vi "TOP LEVEL VI.vi"() -> ()   [LabVIEW 2020]
doc: "This Continuous Measurement sample project is based on the Queued Message Handler template.\n\nThe Event Handling Loop generates messages based on user interface actions.\n\nThe Message Handling Loop processes messages generated by the Event Handling Loop, or by other messages. There are also Acquisition and Logging message handling loop subVIs, and a chart updating loop."
uses:
  Typedefs/Objective selector control enum.ctl
  Typedefs/Laser control knob.ctl
  Typedefs/PMT control knob.ctl
  Typedefs/Frame Size.ctl
  Typedefs/AOL modes.ctl
  Peripherals Control/XYZ Stage/Typedefs/XYZ channel ring.ctl
  Typedefs/Plane Mode.ctl
  Typedefs/AVI implementation enum.ctl
  Acquisition/Typedefs/Ref DAQ Param.ctl
  Typedefs/XY Stage_Move.ctl
  Typedefs/test_fpga_control.ctl
  Typedefs/Reference source.ctl
  User Interface/Typedefs/Laser 1 switch.ctl
  User Interface/Misc/Biology Information.ctl
  User Interface/Misc/Experiment Type.ctl
  Peripherals Control/Laser Ops (Generic)/Type Defs/Ls1 wav cancel.ctl
  Typedefs/Low-High Resolution Settings.ctl
  Typedefs/UI ctrl refs cluster.ctl
  User Interface/Typedefs/Next state queue data.ctl
  Typedefs/Start-Stop Enum.ctl
  Typedefs/Top level VI states.ctl
  Typedefs/Shutter Function Enum.ctl
  <vilib>/Utility/error.llb/DialogType.ctl
  Peripherals Control/Laser Ops (Generic)/Type Defs/Ls1 User Ops.ctl
  Typedefs/fgv_actions.ctl
  Logging/Globals/gl_Binary time series files globals.vi
  Peripherals Control/Pockels/Globals/gl_Pockels control globals.vi
  Global Variables/General Globals.vi
  Peripherals Control/XYZ Stage/Globals/gl_XYZStage globals.vi
  Global Variables/gl_UI Ctrl Refs.vi
  Peripherals Control/XYZ Stage/Typedefs/XYZ stage states.ctl
  Peripherals Control/XYZ Stage/Typedefs/XYZ stage data.ctl
panel:
  out "Camera recording status":bool
  out "Ls1 Status Ind":T1
  in  "Motor Z Stack":bool
  in  "AOL Z Stack":bool
  in  "Live Imaging":bool
  in  "Speed Logging":bool
  in  "Time Lapse":bool
  out "Ls1 wav top Ind":string caption="LASER wavelength"
  out "Ls1 power top Ind":string caption="LASER Output Power"
  in  "Dummy button":bool
  in  "Motor E-Stop":bool
  in  "Movement Correction":bool
  in  "Axis":T2="All" caption="Axis to zero"
  in  "Set as Origin":bool
  out "Stage XYZ Position":cluster{"X":sgl, "Y":sgl, "Z":sgl} caption="Current Stage Position (µm)" {"Z" format="Z:%#_g"; "Y" format="Y:%#_g"; "X" format="X:%#_g"}
  out "Stop":bool=TRUE
  in  "AOL Mode":T3
  in  "Frame Size":T4=512 items=["100X100"=100, "128X128"=128, "200X200"=200, "256X256"=256, "512X512"=512, "1024x1024"=1024, "2048x2048"=2048]
  in  "Objective":T5="Olympus  20X"
  in  "Funct Acq button":bool
  in  "Exit button":bool
  in  "Imaging Param Tab":T6(tab)
  in  "Field of View":sgl(slide)=100.0 min=100 max=500 step=5 scale=100.0..500.0
  in  "AOL Z":sgl(slide) min=-113.4277 max=113.4277 step=0.01 scale=-113.42766999434922..113.42766999434922 scale format="%#_2f"
  in  "PMT 1":T7 max=1000 step=5 scale=0.0..1000.0
  in  "PMT 2":T7 max=1000 step=5 scale=0.0..1000.0
  in  "Zoom":i8(slide)=1 min=1 max=24 step=1 scale=1.0..24.0
  out "Back aperture power (ind.)":dbl format="%#.0fmW"
  in  "Laser Power":T8 caption="LASER" max=1000 step=1 scale=0.0..100.0 scale format="%.0f%"
  out "Power after objective (ind.)":dbl format="%#.0fmW"
  in  "Averages":u16(knob) max=16 step=1 scale=0.0..16.0
  out "Ls1 Note":string
  in  "Dwell Time":dbl=0.10000000149011612 min=0.05 max=12.0 step=0.05000000074505806 format="%#.2fµs"
  in  "Optimise Obj. Pos.":bool=TRUE caption="Optimise Objective Position for AOL Z-stack"
  in  "Obtain Z Stop":bool
  in  "Obtain Z Start":bool
  in  "# Planes":u16=21 min=1 max=1000
  in  "Pockels@Z Stop":u16=5 caption="Laser % at Z Stop" max=100 format="%.0f%"
  in  "Pockels@Z Start":u16=5 caption="Laser % at Z Start" max=100 format="%.0f%"
  in  "Z Step":dbl=2.0 min=0.1 max=500.0 step=0.1 format="%#.1fµm"
  in  "Z Stop":dbl=-25.0 step=1.0 format="%#.0fµm"
  in  "Z Start":dbl=25.0 step=1.0 format="%#.0fµm"
  in  "Ls1 wav cancel":T9
  out "Ls1 Pump peak Hold":bool caption="Laser Pump peak Hold"
  in  "Ls1 Wavelength":dbl caption="Wavelength" format="%#_g [nm]"
  in  "Ls1 Confirm Wav":bool
  out "Ls1 PreChrp Prism2":dbl
  out "Ls1 PreChrp Prism1":dbl caption="Prechirper Prism 1"
  out "Ls1Tuning Status":string caption="Tuning Status"
  out "Ls1 Conn. Status":string caption="Laser Conn. Status"
  out "Ls1 Faults":string caption="Faults"
  out "Ls1 Mode":string caption="Mode"
  in  "Ls1Shutter":bool
  out "Ls1 POWER [mW]":dbl caption="Laser POWER [mW]"
  in  "Hard Shutter":bool
  in  "Virtual Shutter":bool
  out "Center freq ind (nm)":dbl caption="Center frequency" min=800.0 max=1080.0 step=1.0 format="%#.2f MHz"
  out "Ls1 Connection":bool
  in  "Enable f.acq post-processing":bool=TRUE
  in  "Video Record-Funct acq":bool
  in  "Video Record-Live Imaging":bool
  in  "Enable Video Recording":bool
  in  "Plane Mode":T10 items=["XY Plane", "XZ Plane", "YZ Plane", "arbitraryplane"]
  in  "Angle (degrees)":dbl caption="Angle" min=-180.0 max=180.0 format="%#_g°"
  in  "Y centre":dbl min=-1.0 max=1.0 step=0.1 format="%#.2f"
  in  "X centre":dbl min=-1.0 max=1.0 step=0.1 format="%#.2f"
  in  "Live stim.trig.period":dbl=10.0 caption="Stimulus trigger period" min=0.001 max=50.0 step=1.0 format="%#.6f s"
  in  "Live stim.trig.enable":bool caption="Enable stimulus"
  in  "Show ref plots window":bool
  in  "XY Stage Move":T11={"Move"=enum."y_line", "max X displacement"=20.0, "max Y displacement"=20.0, "max speed (um/sec)"=500.0, "Move Stage"=FALSE}
  in  "MovCor Cluster":T12={"x_offset_host"=0.0, "y_offset_host"=0.0, "use host offset"=TRUE, "Set_Ref_Centroid"=FALSE, "OldChirpCode"=FALSE, "use array of offsets"=FALSE, "x_offset_host array"=[], "y_offset_host array "=[], "use host offset Z"=TRUE, "swap Z"=FALSE, "z_offset_host "=0.0} caption="MovCor Setup"
  in  "Target time between mov.cor. ref triggers (ms)":dbl=2.0 caption="Target time between \nmovement correction\nreference triggers (ms)" min=1.0 max=12.0 step=0.1 format="%#_gms"
  in  "Ref Laser Power":u8=12 caption="Ref laser power %" max=100 format="%.0f%"
  out "Pickup mode (ind)":string="<-- From source image"
  in  "RefDAQParam":T13={"Full Frame Size"=0, "Ref Field of View"=0.0, "Ref Zoom"=0, "Ref_dwellTime"=0.0, "Ref X-pixels-per-line(Npxr)"=0, "Ref Y-lines-per-image(Npyr)"=0, "Ref Z-lines-per-image"=0, "Ignore Z lines"=0, "Ref Scan Cycles"=0, "Ref threshold XY"=0, "Ref threshold Z"=1, "Ref average XY"=1, "Ref Average  Z"=0, "Proportional_scale"=1.5999755859375, "Integral_scale"=2047.9375, "Proportional_scale Z"=1.5999755859375, "Integral_scale Z"=400.0, "Diff_threshold"=0.0, "Diff_threshold _z"=0.0, "Sliding Average"=FALSE, "Ref count reset enabled"=TRUE, "Auto-centering"=FALSE} caption="Reference frame DAQ setup" {"Proportional_scale Z" format="%#_15g"; "Ref average XY" min=1 max=64 step=1; "Diff_threshold" format="%#_15g"; "Diff_threshold _z" format="%#_15g"; "Proportional_scale" format="%#_15g"}
  in  "Funct. Acq. Ref frame save":bool
  in  "Reference Source":T14=enum."Red channel"
  in  "Load Reference Image":bool
  in  "Tracking button":bool
  in  "Axial MC":bool
  out "Results Directory Overlay":string
  in  "Paths & Names":T15
  in  "Low-High Resolution Settings":T16={"Resolution low(T)/high(F)"=FALSE, "Three beams(T)/Two beams(F)"=FALSE, "X_only"=FALSE, "Y_only"=FALSE, "Seperation (um)"=1.0, "New Modulation"=FALSE, "Frequency Mix AODs"=FALSE, "Use phase mixed sine"=FALSE, "Prop Low"=0.33, "Prop Mid"=0.33, "Prop High"=0.33} {"Prop High" format="%.2g"; "Prop Mid" format="%.2g"; "Prop Low" format="%.2g"; "Seperation (um)" min=0.0 max=50.0 step=0.01 scale=0.0..50.0}
  in  "Funct. Acq. Pockels Modulation":bool caption="Pockels modulation"
  in  "AVI implementation":T17=enum."AVI2"
  in  "Snapshot":bool
  in  "Generate 3D vol. images":bool caption="Generate 3D vol.\nimages"
  in  "Clear AOL GL":bool
  in  "Abort":bool caption="Stop"
  in  "Experiment Type":T18
  in  "Biology Information":T19
  out "Last State (Ind.)":string
  in  "Switch user":bool
  out "Experiment folder path (ind.)":path caption="Generated experiment folder"
  out "Logging queue (ind)":i32 caption="Elements accumulating\nin the logging queue"
  out "AOL Z-stack Chirps Ready (ind)":bool
  out "Status ind":string
  # "Wavelength [nm]"
  # "Shutters"
  # "Laser Status"
  # "Post-Processing Options"
  # "Cameras Video Recording"
  # "Stimulus Trigger (Live protocols only)"
  # "XY Stage Move"
  # "Reserved for development & debugging only"
  # "Amp. mod. at dF"
  # "New Square Wave"
  # "X1 & Y1"
  # "X2 & Y2"
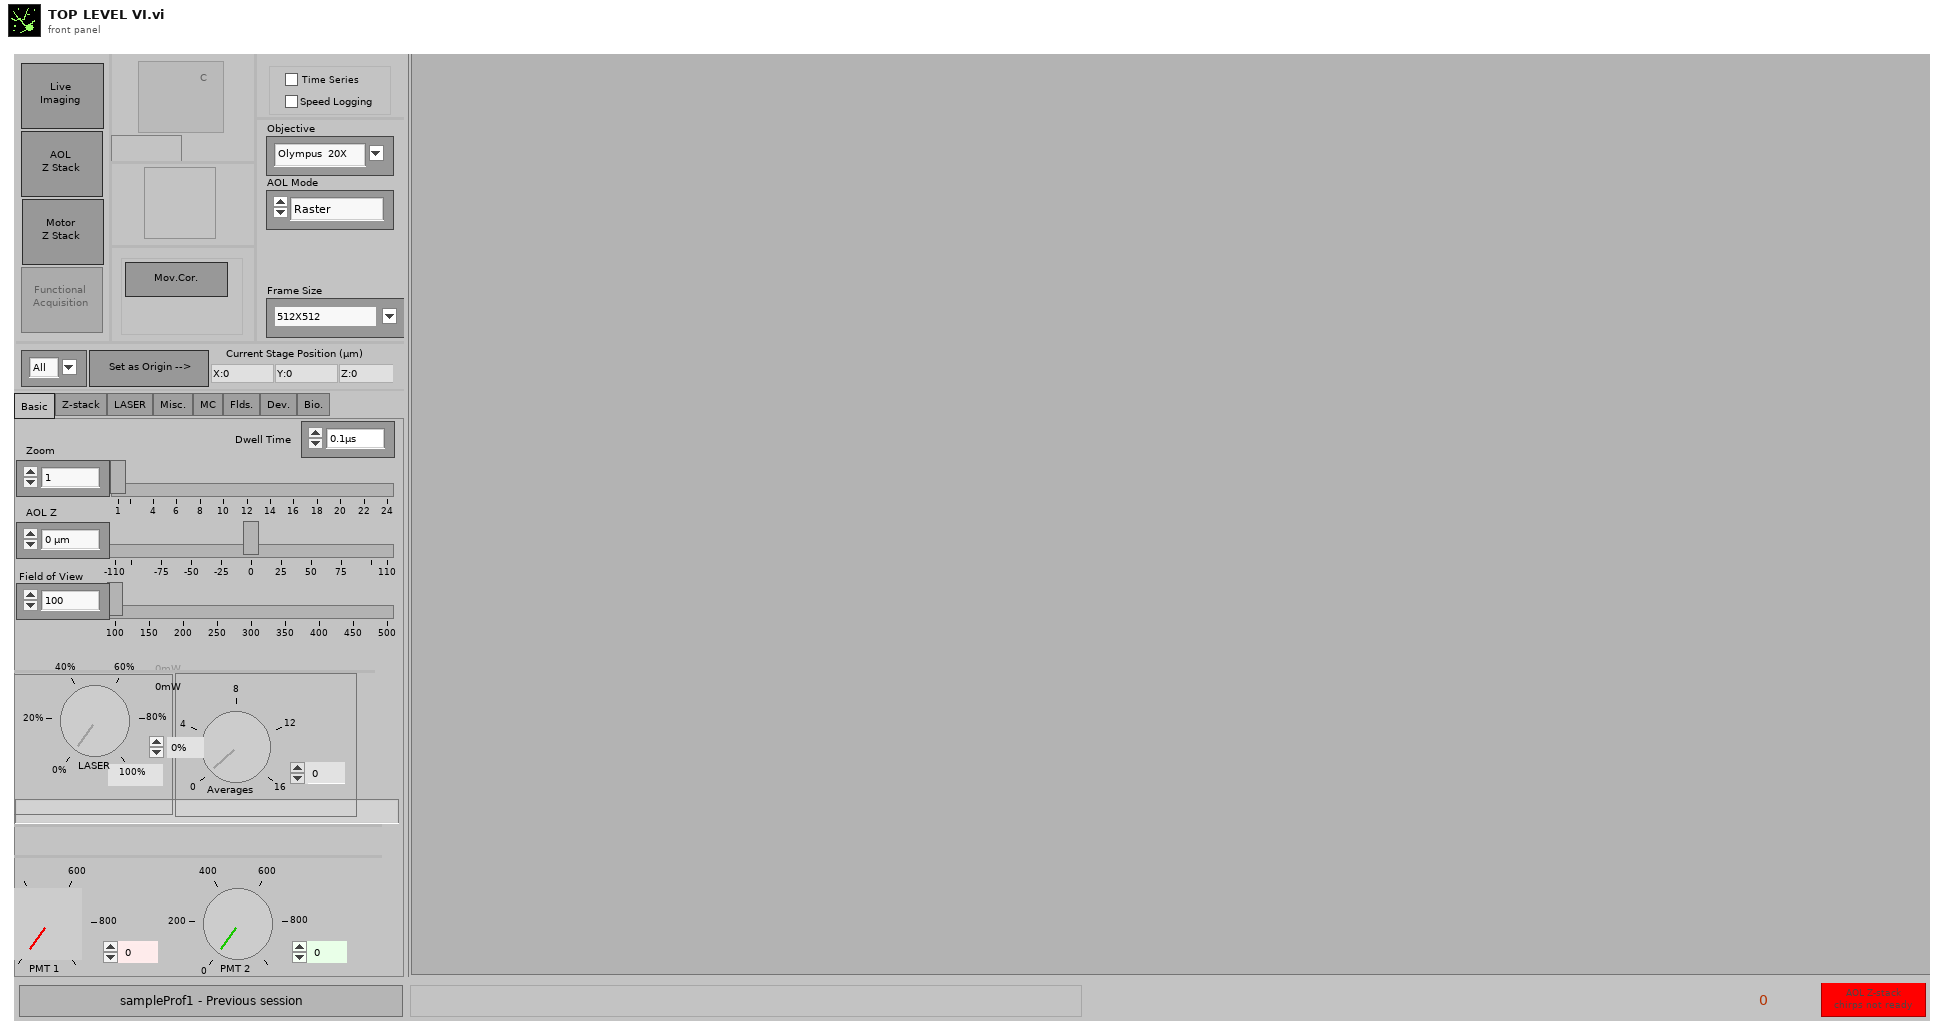
[diagram p1: front panel]
types:
  T1 = typedef "Laser 1 switch.ctl" = bool
  T2 = typedef "XYZ channel ring.ctl" = string
  T3 = typedef "AOL modes.ctl" = enum16{"Raster", "Structural", "Pointing", "Mini Scan", "Alignment"}
  T4 = typedef "Frame Size.ctl" = u16
  T5 = typedef "Objective selector control enum.ctl" = string
  T6 = enum32{"Basic", "Z-stack", "LASER", "Misc.", "MC", "Flds.", "Dev.", "Bio."}
  T7 = typedef "PMT control knob.ctl" = u16
  T8 = typedef "Laser control knob.ctl" = u16
  T9 = typedef "Ls1 wav cancel.ctl" = bool
  T10 = typedef "Plane Mode.ctl" = u16
  T11 = typedef "XY Stage_Move.ctl" = cluster{"Move":enum16{"x-line", "y_line", "x-y-line", "random-xy"}, "max X displacement":sgl, "max Y displacement":sgl, "max speed (um/sec)":sgl, "Move Stage":bool}
  T12 = typedef "test_fpga_control.ctl" = cluster{"x_offset_host":fxp<+/-,16,8>, "y_offset_host":fxp<+/-,16,8>, "use host offset":bool, "Set_Ref_Centroid":bool, "OldChirpCode":bool, "use array of offsets":bool, "x_offset_host array":fxp<+/-,16,8>[], "y_offset_host array ":fxp<+/-,16,8>[], "use host offset Z":bool, "swap Z":bool, "z_offset_host ":fxp<+/-,16,8>}
  T13 = typedef "Ref DAQ Param.ctl" = cluster{"Full Frame Size":u16, "Ref Field of View":sgl, "Ref Zoom":i8, "Ref_dwellTime":sgl, "Ref X-pixels-per-line(Npxr)":i16, "Ref Y-lines-per-image(Npyr)":i16, "Ref Z-lines-per-image":i16, "Ignore Z lines":i16, "Ref Scan Cycles":i32, "Ref threshold XY":u16, "Ref threshold Z":u16, "Ref average XY":u16, "Ref Average  Z":u16, "Proportional_scale":fxp<+,16,2>, "Integral_scale":fxp<+/-,16,12>, "Proportional_scale Z":fxp<+,16,2>, "Integral_scale Z":fxp<+/-,16,12>, "Diff_threshold":fxp<+,16,2>, "Diff_threshold _z":fxp<+,16,2>, "Sliding Average":bool, "Ref count reset enabled":bool, "Auto-centering":bool}
  T14 = typedef "Reference source.ctl" = enum16{"Green channel", "Red channel"}
  T15 = cluster{"Base Directory":path, "User folder?":bool, "Sub-Folder":string, "Experiment folder custom name":string}
  T16 = typedef "Low-High Resolution Settings.ctl" = cluster{"Resolution low(T)/high(F)":bool, "Three beams(T)/Two beams(F)":bool, "X_only":bool, "Y_only":bool, "Seperation (um)":dbl, "New Modulation":bool, "Frequency Mix AODs":bool, "Use phase mixed sine":bool, "Prop Low":dbl, "Prop Mid":dbl, "Prop High":dbl}
  T17 = typedef "AVI implementation enum.ctl" = enum16{"AVI1", "AVI2"}
  T18 = typedef "Experiment Type.ctl" = enum16{"In vivo", "In vitro", "Testing", "Calibration", "Other"}
  T19 = typedef "Biology Information.ctl" = cluster{"Animal Code or Name":string, "Animal DoB":string, "Animal Age":string, "Animal Sex":string, "Animal Weight":string, "Date of Injection":string, "Date of Implant":string, "Site of Injection":string, "Animal Ear Notch":string, "AAV constructs":string, "Genetic background":string, "Optical reporter":string, "Region of brain imaged":string, "Other \ncomments":string}
  T20 = enum8{"Enabled", "Disabled", "Disabled and Grayed Out"}
  T21 = typedef "Next state queue data.ctl" = cluster{"Start/Stop":T22, "State":T23}
  T22 = typedef "Start-Stop Enum.ctl" = enum16{"START", "STOP"}
  T23 = typedef "Top level VI states.ctl" = enum16{"None", "Initialise UI", "<STACK PROTOCOL STATES>", "AOL Zstack-START", "AOL Zstack-STOP", "Motor Zstack-START", "Motor Zstack-STOP", "Parameter Sweep-START", "Parameter Sweep-STOP", "<ACQUISITION PROTOCOL STATES> ", "Functional Acquisition-START", "Functional Acquisition-STOP", "Single Plane Acquisition-START", "Single Plane Acquisition-STOP", "Volume Acquisition-START", "Volume Acquisition-STOP", "<LIVE IMAGING PROTOCOL STATES>", "Live Imaging-START", "Live Imaging-STOP", "Live Plane Imaging-START", "Live Plane Imaging-STOP", "Live Volume Imaging-START", "Live Volume Imaging-STOP", "<MOVEMENT CORRECTION PROTOCOL STATES>", "EXIT"}
  T24 = enum16{"Start", "Display status", "Monitor", "Cancel", "Stop"}
  T25 = enum16{"Write Red AVI", "Write Green AVI", "Write AVI mode"}
  T26 = typedef "Shutter Function Enum.ctl" = enum16{"Open Shutter", "Close Shutter"}
  T27 = typedef "XYZ stage data.ctl" = cluster{"Command":T28, "Channel":T2, "X":sgl, "Y":sgl, "Z":sgl, "Speed":i32, "Zero":bool, "Use acknowledgement?":bool}
  T28 = typedef "XYZ stage states.ctl" = enum16{"Dequeue", "Initialize", "Read Position", "Read Speed Setting", "Move", "Set Max Speed", "Reset Axis", "Stop all movement"}
  T29 = typedef "Ls1 User Ops.ctl" = enum16{"Setup", "Initialise", "Disable Controls", "Enable Controls", "Update Connection Info", "Update Laser Warning", "Update Laser status", "Update Laser status - sel", "Update Laser Wav.", "Update Laser Power", "Update prechiper settings", "Update Laser Note", "Update Shutter Status", "Close"}
  T30 = typedef "fgv_actions.ctl" = enum16{"Get", "Set"}
  T31 = enum16{"Software Init", "User menu", "Switch User button"}
  T32 = typedef "UI ctrl refs cluster.ctl" = cluster{"Top level VI path":path, "Top level VI ref":refnum<vi>, "User menu ref":refnum<k9>, "Sub Panel control":refnum<vi>, "Imaging Param Tab":refnum<vi>, "Occurrence-Start drivers":refnum<k4>, "Occurrence-Speed logging initialised":refnum<k4>, "Occurrence-XYZ stage initialised":refnum<k4>, "Exit button":refnum<vi>, "Status ind":refnum<vi>, "Set as origin":refnum<vi>, "Speed Logging":refnum<vi>, "Time Lapse":refnum<vi>, "Live Imaging":refnum<vi>, "AOL Z Stack":refnum<vi>, "Motor Z Stack":refnum<vi>, "Funct Acq button":refnum<vi>, "Hard Shutter":refnum<vi>, "Virtual Shutter":refnum<vi>, "Laser Power":refnum<vi>, "AOL Mode":refnum<vi>, "Frame Size":refnum<vi>, "Field of View":refnum<vi>, "Dwell Time":refnum<vi>, "Zoom":refnum<vi>, "AOL Z":refnum<vi>, "Objective":refnum<vi>, "Axis":refnum<vi>, "Paths & Names":refnum<vi>, "Experiment folder path (ind.)":refnum<vi>, "Last State (Ind.)":refnum<vi>, "Averages":refnum<vi>, "Angle (degrees)":refnum<vi>, "X centre":refnum<vi>, "Y centre":refnum<vi>, "Plane Mode":refnum<vi>, "# Planes":refnum<vi>, "Z Start":refnum<vi>, "Z Stop":refnum<vi>, "Z Step":refnum<vi>, "PMT 1":refnum<vi>, "PMT 2":refnum<vi>, "Stage XYZ Position":refnum<vi>, "Pockels@Z Start":refnum<vi>, "Pockels@Z Stop":refnum<vi>, "Obtain Z Start":refnum<vi>, "Obtain Z Stop":refnum<vi>, "Live stim.trig.period":refnum<vi>, "Live stim.trig.enable":refnum<vi>, "Movement Correction":refnum<vi>, "Load Reference Image":refnum<vi>, "XY Stage Move":refnum<vi>, "MovCor Cluster":refnum<vi>, "RefDAQParam":refnum<vi>, "Funct. Acq. Pockels Modulation":refnum<vi>, "Ref Laser Power":refnum<vi>, "Enable Video Recording":refnum<vi>, "Video Record-Live Imaging":refnum<vi>, "Video Record-Funct acq":refnum<vi>, "Reference Source":refnum<vi>, "AOL Z-stack Chirps Ready (ind)":refnum<vi>, "Target time between mov.cor. ref triggers (ms)":refnum<vi>, "Funct. Acq. Ref frame save":refnum<vi>, "Tracking button":refnum<vi>, "Show ref plots window":refnum<vi>, "Center freq ind (nm)":refnum<vi>, "Pickup mode (ind)":refnum<vi>, "Logging queue (ind)":refnum<vi>, "Back aperture power (ind.)":refnum<vi>, "Power after objective (ind.)":refnum<vi>, "Switch user":refnum<vi>, "Ls1 Conn. Status":refnum<vi>, "Ls1Tuning Status":refnum<vi>, "Ls1 Faults":refnum<vi>, "Ls1 Connection":refnum<vi>, "Ls1 Mode":refnum<vi>, "Ls1 POWER [mW]":refnum<vi>, "Ls1Shutter":refnum<vi>, "Ls1 Wavelength":refnum<vi>, "Ls1 Note":refnum<vi>, "Ls1 Confirm Wav":refnum<vi>, "Ls1 PreChrp Prism1":refnum<vi>, "Ls1 PreChrp Prism2":refnum<vi>, "Ls1 wav top Ind":refnum<vi>, "Ls1 power top Ind":refnum<vi>, "Ls1 Pump peak Hold":refnum<vi>, "Ls1 Status Ind":refnum<vi>, "Ls1 wav cancel":refnum<vi>, "Experiment Type":refnum<vi>, "Biology Information":refnum<vi>, "Camera recording status":refnum<vi>, "Optimise Obj. Pos.":refnum<vi>}
  T33 = typedef "All Message Queues.ctl" = cluster{"UI queue":refnum<queue>, "Acq. queue":refnum<queue>, "Logging queue":refnum<queue>}
  T34 = typedef "DialogType.ctl" = u16
  T35 = typedef "AOL_Globals.ctl" = cluster{"Imaging Protocol":T36, "Number of POI":u16, "Number of Miniscans":u16, "Number of Trials":u16, "Number of Cycles ":u64, "# Averaged Frames":u16, "Laser power (%)":u8, "Pockels (V)":dbl, "Acquisition Length (sec)":dbl, "Fill time (us)":dbl, "POI Dwell time (us)":dbl, "Miniscan Dwell time per pixel (us)":dbl, "PMT 1":dbl, "PMT 2":dbl, "Back Apperture (mA)":dbl, "Frame Size":T4, "Center Frequency":dbl, "Field of View (um)":dbl, "Field of View (norm)":dbl, "DwellTime (us)":dbl, "Ref Dwell Time (us)":dbl, "Wavelength (nm)":dbl, "Zoom":dbl, "AOL Z":dbl, "AOL Mode":T3, "GridXY":dbl, "GridZ":dbl, "TriggerPeriod (sec)":dbl, "Number of Pixels in Miniscan":u16, "Experiment folder path":path, "X centre":dbl, "Y centre":dbl, "Angle (degrees)":dbl, "Angle Xs (degrees)":dbl, "Angle Ys (degrees)":dbl, "Plane Mode":T10, "Threshold":u16[], "Regenerate Chirps":bool, "Rectangle ROI length (pixels)":u16, "Rectangle ROI height (pixels)":u16, "AOD fill":u16, "StartupDelay":i32, "Samples Wait after Trigger":u16, "Slip Cycle":u32, "Add Cycle":bool, "Functional Mode":T37, "Z Start":dbl, "Z Stop":dbl, "# Planes":i32, "Total Pixels":i32, "Variable Miniscan Pixels":u16[], "Use Variable Length":bool, "Use Variable Resolution":bool, "Laser power (%) at Z Start":u8, "Laser power (%) at Z Stop":u8, "Ref Z Step":i8}
  T36 = typedef "Imaging Protocols enum.ctl" = enum16{"AOL Z-Stack", "Motor Z Stack", "Parameter Sweep", "Functional Acquisition", "Single Plane Acquisition", "Volume Acquisition", "Live Imaging", "Live Plane Imaging", "Live Volume Imaging"}
  T37 = typedef "Functional Mode.ctl" = enum16{"Point", "Line", "Patch", "Plane", "Volume"}
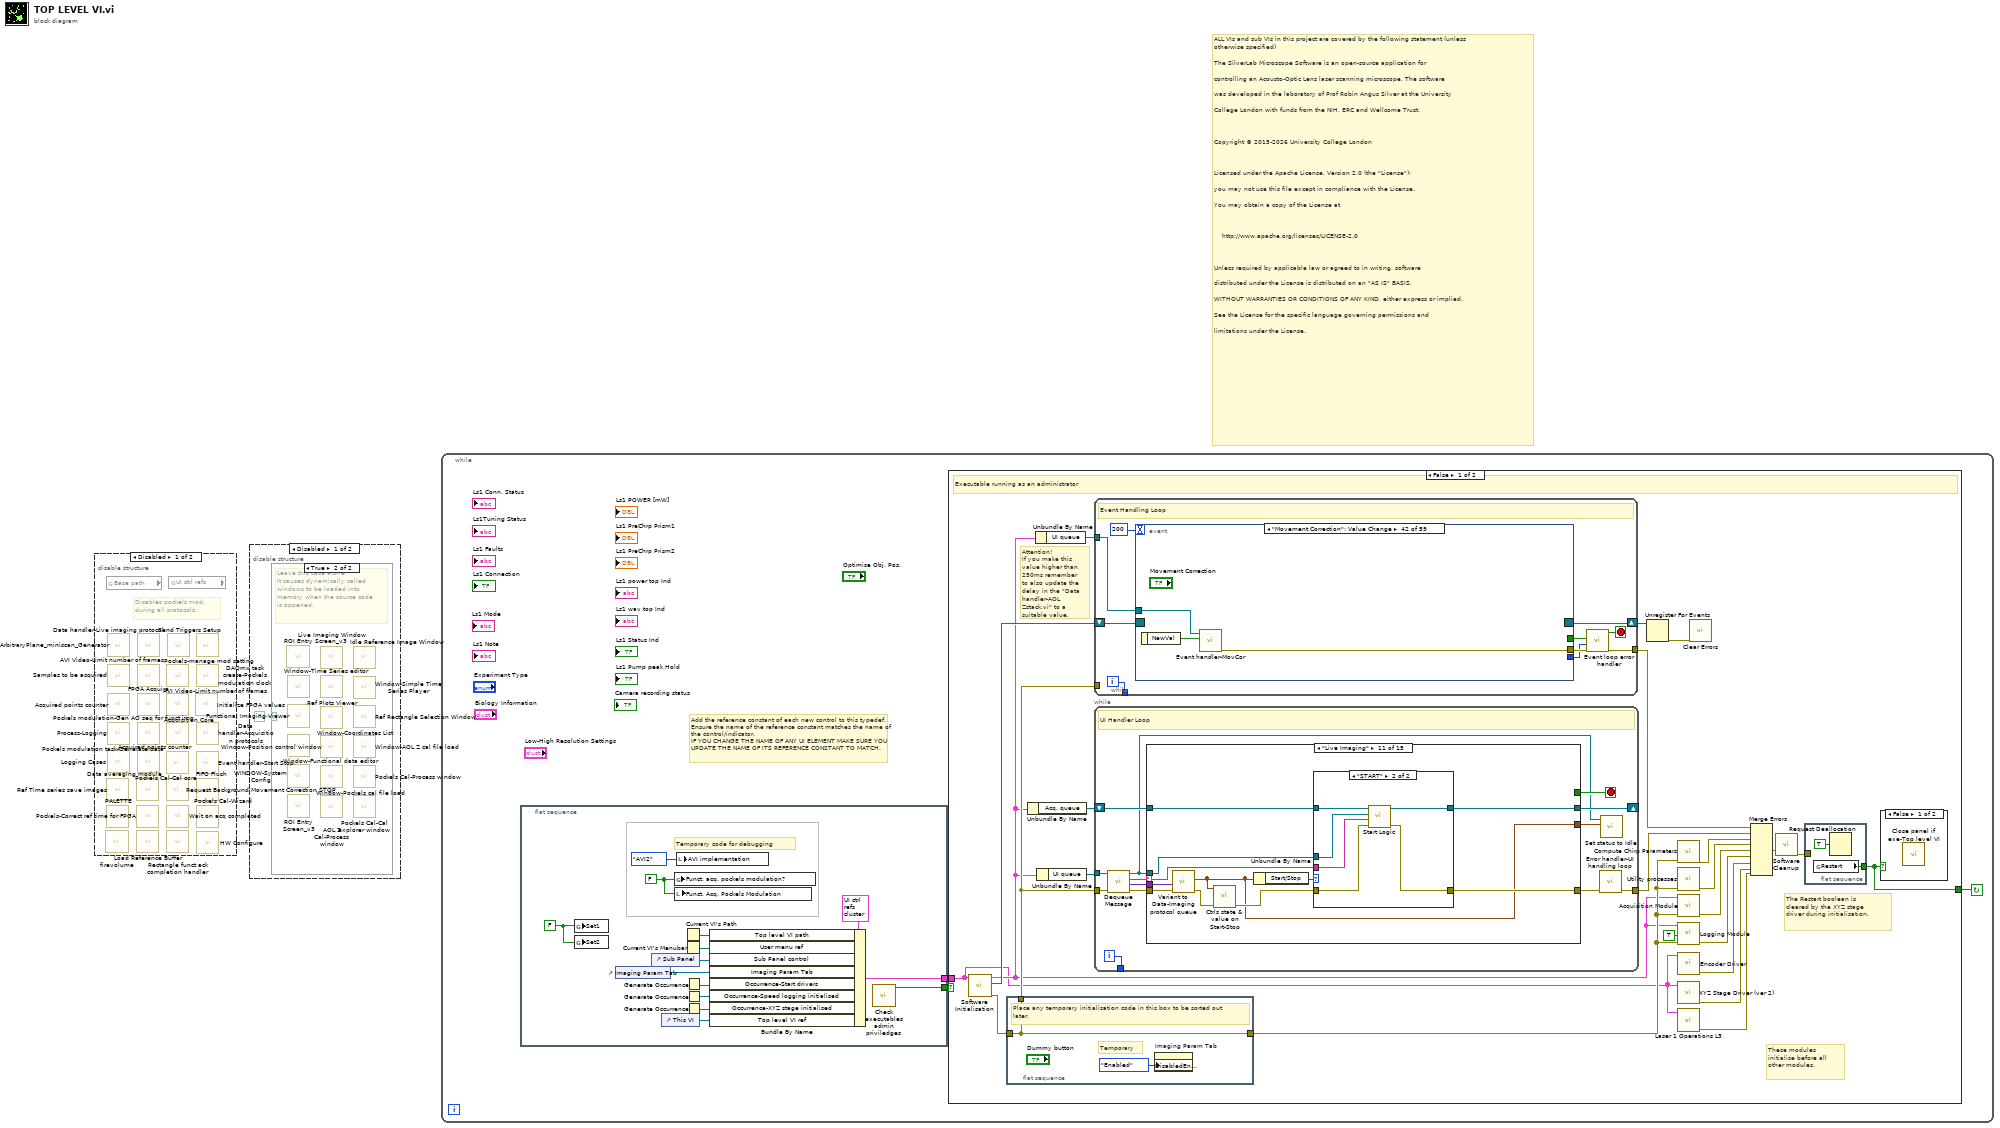
[diagram p0: block diagram]
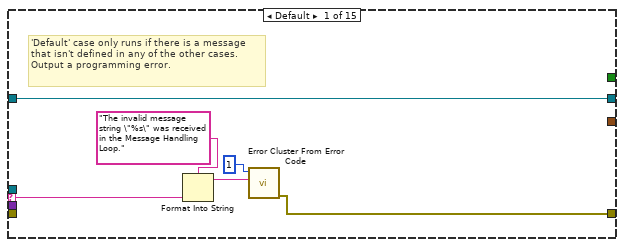
[diagram p5: hidden frame]
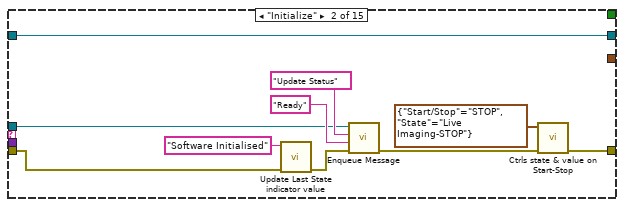
[diagram p6: hidden frame]
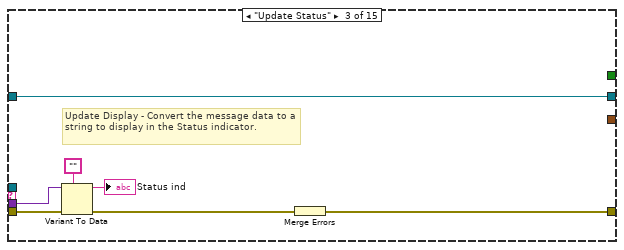
[diagram p7: hidden frame]
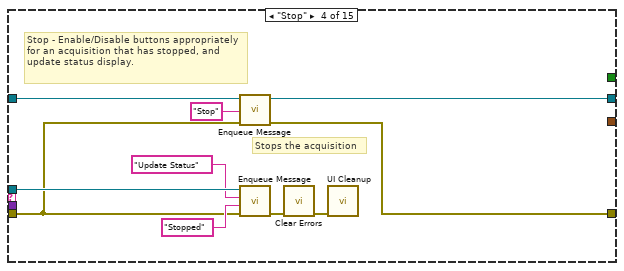
[diagram p8: hidden frame]
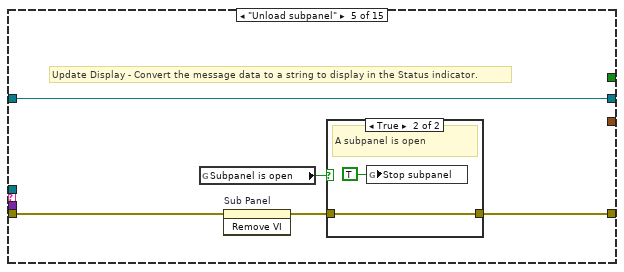
[diagram p9: hidden frame]
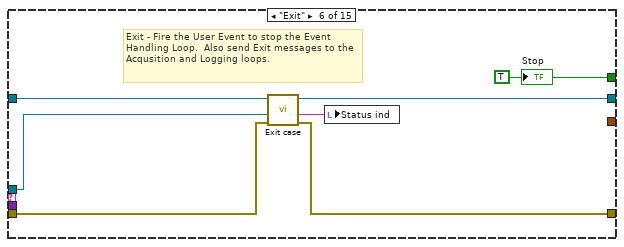
[diagram p11: hidden frame]
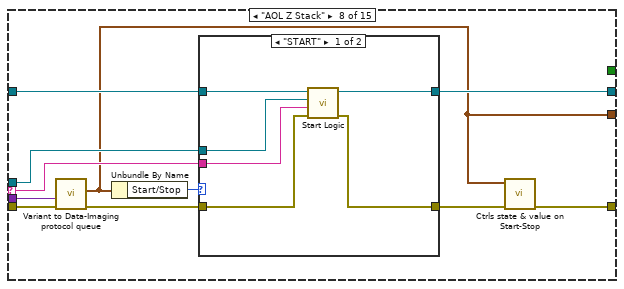
[diagram p13: hidden frame]
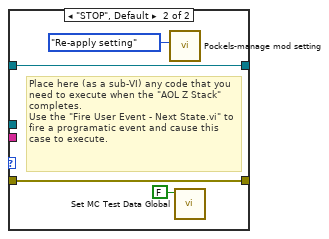
[diagram p14: hidden frame]
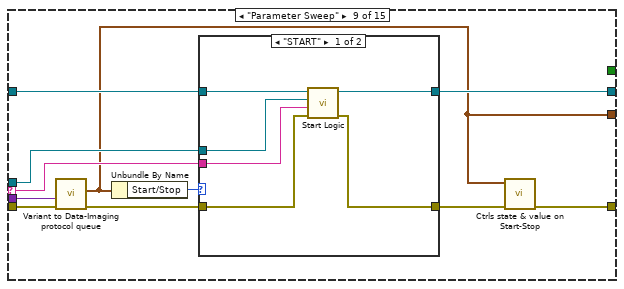
[diagram p15: hidden frame]
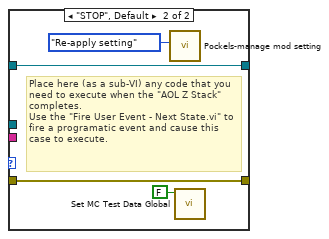
[diagram p16: hidden frame]
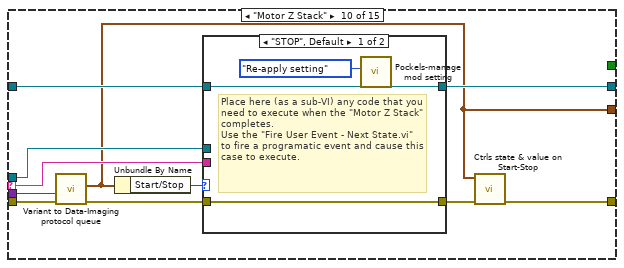
[diagram p17: hidden frame]
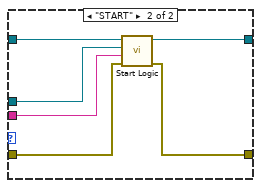
[diagram p18: hidden frame]
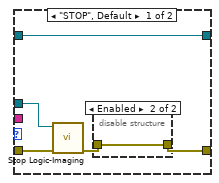
[diagram p19: hidden frame]
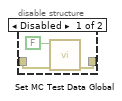
[diagram p20: hidden frame]
diagram:
  # "ALL VIs and sub VIs in this project are covered by the following statement (unless \notherwise specified)\n\nThe SilverLab Microscope Software is an open-source application for\n\ncontrolling an Acousto-Optic Lens laser scanning microscope. The software\n\nwas developed in the laboratory of Prof Robin Angus Silver at the University\n\nCollege London with funds from the NIH, ERC and Wellcome Trust.\n\n \n\nCopyright © 2015-2026 University College London\n\n \n\nLicensed under the Apache License, Version 2.0 (the \"License\");\n\nyou may not use this file except in compliance with the License.\n\nYou may obtain a copy of the License at\n\n \n\n    http://www.apache.org/licenses/LICENSE-2.0\n\n \n\nUnless required by applicable law or agreed to in writing, software\n\ndistributed under the License is distributed on an \"AS IS\" BASIS,\n\nWITHOUT WARRANTIES OR CONDITIONS OF ANY KIND, either express or implied.\n\nSee the License for the specific language governing permissions and\n\nlimitations under the License."
  n1 = disable-structure shown="Disabled" {
    frame Disabled {
      # "Disables pockels mod.\nduring all protocols."
      n2 = call "firevolume.vi"() -> ()  [unwired: 12 in]
      n3 = global read "General Globals.vi" "Base path"() -> ()  [unwired: 1 out]
      n4 = call "Ref Time series save images.vi"() -> ()  [unwired: 11 in, 1 out]
      n5 = call "PALETTE.vi"() -> ()  [unwired: 12 in]
      n6 = call "ArbitraryPlane_miniscan_Generator.vi"() -> ()  [unwired: 7 in, 5 out]
      n7 = call "Samples to be acquired.vi"() -> ()  [unwired: 9 in, 3 out]
      n8 = call "Acquired points counter.vi"() -> ()  [unwired: 12 in, 4 out]
      n9 = call "Process-Logging.vi"() -> ()  [unwired: 11 in, 1 out]
      n10 = call "Logging Cases.vi"() -> ()  [unwired: 14 in, 2 out]
      n11 = call "Data averaging module.vi"() -> ()  [unwired: 5 in, 7 out]
      n12 = call "Pockels-Correct ref time for FPGA.vi"() -> ()  [unwired: 10 in, 2 out]
      n13 = call "Load Reference Buffer.vi"() -> ()  [unwired: 11 in, 1 out]
      n14 = call "Data handler-Live imaging protocol.vi"() -> ()  [unwired: 15 in, 1 out]
      n15 = call "AVI Video-Limit number of frames.vi"() -> ()  [unwired: 1 in, 1 out]
      n16 = call "FPGA Acquire.vi"() -> ()  [unwired: 11 in, 5 out]
      n17 = call "Pockels modulation task-Generate data.vi"() -> ()  [unwired: 7 in, 5 out]
      n18 = call "Pockels Cal-Cal core.vi"() -> ()  [unwired: 9 in, 3 out]
      n19 = call "Acquired points counter.vi"() -> ()  [unwired: 12 in, 4 out]
      n20 = call "Request Background Movement Correction STOP.vi"() -> ()  [unwired: 10 in, 2 out]
      n21 = call "AVI Video-Limit number of frames.vi"() -> ()  [unwired: 1 in, 1 out]
      n22 = call "Acquisition Core.vi"() -> ()  [unwired: 10 in, 2 out]
      n23 = call "Pockels modulation-Gen AO seq for funct img.vi"() -> ()  [unwired: 8 in, 4 out]
      n24 = call "Wait on acq completed.vi"() -> ()  [unwired: 11 in, 1 out]
      n25 = call "Rectangle funct ack completion handler.vi"() -> ()  [unwired: 12 in]
      n26 = call "Pockels-manage mod setting.vi"() -> ()  [unwired: 11 in, 1 out]
      n27 = global read "gl_UI Ctrl Refs.vi" "UI ctrl refs"() -> ()  [unwired: 1 out]
      n28 = call "Initialize FPGA values.vi"() -> ()  [unwired: 10 in, 2 out]
      n29 = call "Send Triggers Setup.vi"() -> ()  [unwired: 10 in, 2 out]
      n30 = call "DAQmx task create-Pockels modulation clock.vi"() -> ()  [unwired: 10 in, 2 out]
      n31 = call "Data handler-Acquisition protocols.vi"() -> ()  [unwired: 14 in, 2 out]
      n32 = call "Event handler-Start Stop.vi"() -> ()  [unwired: 10 in, 2 out]
      n33 = call "FIFO Flush.vi"() -> ()  [unwired: 9 in, 3 out]
      n34 = call "Pockels Cal-Wizard.vi"() -> ()  [unwired: 12 in]
      n35 = call "HW Configure.vi"() -> ()  [unwired: 10 in, 2 out]
    }
    frame Enabled {
    }
  }
  n36 = disable-structure shown="Disabled" {
    frame Disabled {
      n37 = case shown="True" FALSE {
        frame False {
        }
        frame True {
          # "Leave this case alone.\nIt causes dynamically called windows to be loaded into memory when the source code is oppened."
          n38 = call "ROI Entry Screen_v3.vi"() -> ()  [unwired: 12 in]
          n39 = call "Window-Time Series editor.vi"() -> ()  [unwired: 12 in]
          n40 = call "Functional Imaging Viewer.vi"() -> ()  [unwired: 12 in]
          n41 = call "Window-Functional data editor.vi"() -> ()  [unwired: 12 in]
          n42 = call "WINDOW-System Config.vi"() -> ()  [unwired: 12 in]
          n43 = call "ROI Entry Screen_v3.vi"() -> ()  [unwired: 12 in]
          n44 = call "Live Imaging Window.vi"() -> ()  [unwired: 12 in]
          n45 = call "Ref Plots Viewer.vi"() -> ()  [unwired: 12 in]
          n46 = call "Window-Coordinates List.vi"() -> ()  [unwired: 12 in]
          n47 = call "Window-Position control window.vi"() -> ()  [unwired: 12 in]
          n48 = call "Window-Pockels cal file load.vi"() -> ()  [unwired: 12 in]
          n49 = call "AOL Z Cal-Process window.vi"() -> ()  [unwired: 9 in, 3 out]
          n50 = call "Idle Reference Image Window.vi"() -> ()  [unwired: 12 in]
          n51 = call "Window-Simple Time Series Player.vi"() -> ()  [unwired: 12 in]
          n52 = call "Ref Rectangle Selection Window.vi"() -> ()  [unwired: 10 in, 2 out]
          n53 = call "Window-AOL Z cal file load.vi"() -> ()  [unwired: 12 in]
          n54 = call "Pockels Cal-Process window.vi"() -> ()  [unwired: 10 in, 2 out]
          n55 = call "Pockels Cal-Cal explorer window.vi"() -> ()  [unwired: 12 in]
        }
      }
    }
    frame Enabled {
    }
  }
  n56 = while {
    stop <- w4 continue-if-true
    # "Add the reference constant of each new control to this typedef. Ensure the name of the reference constant matches the name of the control/indicator.\nIF YOU CHANGE THE NAME OF ANY UI ELEMENT MAKE SURE YOU UPDATE THE NAME OF ITS REFERENCE CONSTANT TO MATCH."
    n57 = flat-sequence {
      tunnel: [w426] -> w3
      tunnel: [w415] -> w2
      frame #0 {
        w414 = FALSE ("Funct. acq. pockels modulation?")
        w419 = FALSE ("Set1")
        # "Temporary code for debugging"
        n58 = global write "gl_Binary time series files globals.vi" "Set1"(w419) -> ()
        n59 = global write "gl_Binary time series files globals.vi" "Set2"(w419) -> ()
        n60 = control-ref of="Imaging Param Tab"() -> (w413:refnum<vi>)
        n61 = control-ref of="Sub Panel"() -> (w416:refnum<vi>)
        n62 = control-ref of="This VI"() -> (w420:refnum<vi>)
        n63 = global write "gl_Pockels control globals.vi" "Funct. acq. pockels modulation?"(w414) -> ()
        n64 = local write "Funct. Acq. Pockels Modulation"(w414) -> ()
        n65 = local write "AVI implementation"(AVI_implementation_enum."AVI2" ("AVI implementation")) -> ()
        n66 = Current VI's Path() -> (path=w424:path)
        n67 = Current VI's Menubar() -> (w425:refnum<k9>)
        n68 = Generate Occurrence() -> (w417:refnum<k4>)
        n69 = Generate Occurrence() -> (w421:refnum<k4>)
        n70 = Generate Occurrence() -> (w422:refnum<k4>)
        n71 = Bundle By Name(cluster=T32 {"Top level VI path"=path "", "Top level VI ref"=refnum, "User menu ref"=refnum, "Sub Panel control"=refnum, "Imaging Param Tab"=refnum, "Occurrence-Start drivers"=refnum, "Occurrence-Speed logging initialised"=refnum, "Occurrence-XYZ stage initialised"=refnum, "Exit button"=refnum, "Status ind"=refnum, "Set as origin"=refnum, "Speed Logging"=refnum, "Time Lapse"=refnum, "Live Imaging"=refnum, "AOL Z Stack"=refnum, "Motor Z Stack"=refnum, "Funct Acq button"=refnum, "Hard Shutter"=refnum, "Virtual Shutter"=refnum, "Laser Power"=refnum, "AOL Mode"=refnum, "Frame Size"=refnum, "Field of View"=refnum, "Dwell Time"=refnum, "Zoom"=refnum, "AOL Z"=refnum, "Objective"=refnum, "Axis"=refnum, "Paths & Names"=refnum, "Experiment folder path (ind.)"=refnum, "Last State (Ind.)"=refnum, "Averages"=refnum, "Angle (degrees)"=refnum, "X centre"=refnum, "Y centre"=refnum, "Plane Mode"=refnum, "# Planes"=refnum, "Z Start"=refnum, "Z Stop"=refnum, "Z Step"=refnum, "PMT 1"=refnum, "PMT 2"=refnum, "Stage XYZ Position"=refnum, "Pockels@Z Start"=refnum, "Pockels@Z Stop"=refnum, "Obtain Z Start"=refnum, "Obtain Z Stop"=refnum, "Live stim.trig.period"=refnum, "Live stim.trig.enable"=refnum, "Movement Correction"=refnum, "Load Reference Image"=refnum, "XY Stage Move"=refnum, "MovCor Cluster"=refnum, "RefDAQParam"=refnum, "Funct. Acq. Pockels Modulation"=refnum, "Ref Laser Power"=refnum, "Enable Video Recording"=refnum, "Video Record-Live Imaging"=refnum, "Video Record-Funct acq"=refnum, "Reference Source"=refnum, "AOL Z-stack Chirps Ready (ind)"=refnum, "Target time between mov.cor. ref triggers (ms)"=refnum, "Funct. Acq. Ref frame save"=refnum, "Tracking button"=refnum, "Show ref plots window"=refnum, "Center freq ind (nm)"=refnum, "Pickup mode (ind)"=refnum, "Logging queue (ind)"=refnum, "Back aperture power (ind.)"=refnum, "Power after objective (ind.)"=refnum, "Switch user"=refnum, "Ls1 Conn. Status"=refnum, "Ls1Tuning Status"=refnum, "Ls1 Faults"=refnum, "Ls1 Connection"=refnum, "Ls1 Mode"=refnum, "Ls1 POWER [mW]"=refnum, "Ls1Shutter"=refnum, "Ls1 Wavelength"=refnum, "Ls1 Note"=refnum, "Ls1 Confirm Wav"=refnum, "Ls1 PreChrp Prism1"=refnum, "Ls1 PreChrp Prism2"=refnum, "Ls1 wav top Ind"=refnum, "Ls1 power top Ind"=refnum, "Ls1 Pump peak Hold"=refnum, "Ls1 Status Ind"=refnum, "Ls1 wav cancel"=refnum, "Experiment Type"=refnum, "Biology Information"=refnum, "Camera recording status"=refnum, "Optimise Obj. Pos."=refnum} ("output cluster"), "Top level VI path"=w424, "User menu ref"=w425, "Sub Panel control"=w416, "Imaging Param Tab"=w413, "Occurrence-Start drivers"=w417, "Occurrence-Speed logging initialised"=w421, "Occurrence-XYZ stage initialised"=w422, "Top level VI ref"=w420) -> (w426:T32)
        n72 = call "Check executables admin priviledges.vi"() -> ("Exe not run as an administrator"=w415:bool)  [unwired: 10 in, 1 out]
      }
    }
    n73 = case shown="False" w2 {
      tunnel: [w26 FALSE ("Restart")] -> w4
      tunnel: w3 -> [w5 w411]
      frame False {
        # "The Restart boolean is cleared by the XYZ stage driver during initialisation."
        # "These modules initialise before all other modules."
        # "Attention!\nIf you make this value higher than 250ms remember to also update the delay in the \"Data handler-AOL Zstack.vi\" to a suitable value."
        # "Executable running as an administrator"
        n74 = call "Software Initialisation.vi"("UI elements cluster"=w5) -> ("Error Out"=w27:errorcluster, "Event Registration Refnum"=w28:refnum<event-registration>, "Message Queues out"=w7:T33)  [unwired: 8 in]
        n75 = flat-sequence {
          tunnel: w27 -> [w31]
          tunnel: [w31] -> w11
          tunnel: [w31] -> w10
          frame #0 {
            # "Temporary"
            # "Place any temporary initialisation code in this box to be sorted out later."
            n76 = property on="Imaging Param Tab" class="TabCtl (strict)"("DisabledEnum"=T20."Enabled" ("Disabled")) -> ()  [unwired: 2 in, 2 out]
          }
        }
        n77 = Unbundle By Name(w7) -> ("Acq. queue"=w22:refnum<queue>)
        n78 = Unbundle By Name(w7) -> ("UI queue"=w24:refnum<queue>)
        n79 = Unbundle By Name(w7) -> ("UI queue"=w23:refnum<queue>)
        n80 = while {
          tunnel: w24 -> [w272]
          tunnel: [w270] -> w15
          shift-right: [w271] -> w25
          shift-left: w28 -> [w273]
          tunnel: [w267] -> _
          tunnel: w11 -> [_]
          i -> [w267]
          stop <- w275 stop-if-true
          # "Event Handling Loop"
          n81 = event shown="[41] \"Movement Correction\": Value Change" {
            selector: w273 -> [_ _ _ _ _ _ _ _ _ _ _ _ _ _ _ _ _ _ _ _ _ _ _ _ _ _ _ _ _ _ _ _ _ _ _ _ _ _ _ _ _ _ _ _ _ _ _ _ _ _ _ _ _ _ _ _ _ _ _]
            dyn-events: [_ _ _ _ _ _ _ _ _ _ _ _ _ _ _ _ _ _ _ _ _ _ _ _ _ _ _ _ _ _ _ _ _ _ _ _ _ _ _ _ _ _ _ _ _ _ _ _ _ _ _ _ _ _ _ _ _ _ _] -> w271
            timeout: 200 -> [_ _ _ _ _ _ _ _ _ _ _ _ _ _ _ _ _ _ _ _ _ _ _ _ _ _ _ _ _ _ _ _ _ _ _ _ _ _ _ _ _ _ _ _ _ _ _ _ _ _ _ _ _ _ _ _ _ _ _]
            tunnel: [_ _ _ _ _ _ _ _ _ _ _ _ _ _ _ _ _ _ _ _ _ _ _ _ _ _ _ _ _ _ _ _ _ _ _ _ _ _ _ _ _ _ _ _ _ _ _ _ _ _ _ _ _ _ _ _ TRUE ("Discard?") _ _] -> w268
            tunnel: w272 -> [_ w278 _ _ w283 _ _ _ _ _ _ _ _ _ _ _ _ _ _ _ _ _ _ _ _ _ _ _ _ _ _ _ _ _ _ _ _ _ _ _ _ w346 _ _ _ _ _ _ _ _ _ _ _ _ _ w403 _ w406 w409]
            tunnel: [_ w277 _ _ w282 _ _ _ _ w289 w294 w296 w298 _ _ w302 _ _ _ _ _ _ _ _ _ _ _ _ _ _ _ _ _ _ _ _ _ _ _ _ w343 w344 _ _ _ _ _ _ w392 _ _ _ _ _ _ w402 _ w407 w410] -> w274
            tunnel: [_ _ _ _ w281 _ _ _ _ _ _ _ _ _ _ _ _ _ _ _ _ _ _ _ _ _ _ _ _ _ _ _ _ _ _ _ _ _ _ _ _ _ _ _ _ _ _ _ _ _ _ _ _ _ _ _ _ _ _] -> w266
            event Timeout {
              n82 = event-data() -> ()  [unwired: 1 in, 1 out]
              n83 = call "monitor wavelength change.vi"("Actions"=T24."Monitor") -> ()  [unwired: 8 in, 3 out]
            }
            event Menu Selection (User); "Experiment folder path (ind.)", "Results Directory Overlay": Shortcut Menu Selection (User) {
              n84 = event-data() -> ("ItemTag"=w279:string)  [unwired: 1 in]
              n85 = call "User menu handler.vi"("UI queue"=w278, "User Menu ItemTag"=w279) -> ("error out"=w277:errorcluster)  [unwired: 9 in]
            }
            event "Live stim.trig.period", "Set as Origin", "Stage XYZ Position.X", "Stage XYZ Position.Y", "Stage XYZ Position.Z": Shortcut Menu Selection (User) {
              n86 = event-data() -> ("ItemTag"=w280:string)  [unwired: 1 in]
              n87 = call "Top level UI-Shortcut menus handler.vi"("ItemTag"=w280) -> ()  [unwired: 11 in]
            }
            event Menu Activation? {
              n88 = event-data() -> ()  [unwired: 1 in, 5 out]
              n89 = call "menu-Cal group disabled state.vi"() -> ()  [unwired: 10 in, 2 out]
              n90 = event-data() -> ()  [unwired: 2 in, 1 out]
            }
            event User Event {
              # "Causes the \"UI Handler Loop\" to execute one of its cases. There are redundant cases as a provision.\nThis functionality is fully scalable and flexible allowing to programatically fire events from anywhere within the software, as well as when the user presses a button.\nThis event case also executes in response to a programmatic event which occurs when the user closes the ROI Entry Screen, and executes the required case, depending on which button the user pressed to exit the ROI Entry Screen."
              n91 = event-data() -> ("Next State"=w281:T23)  [unwired: 1 in]
              n92 = call "Event handler-Start Stop.vi"("Next State"=w281, "UI queue"=w283) -> ("error out"=w282:errorcluster)  [unwired: 8 in, 1 out]
            }
            event "Experiment folder path (ind.)": Shortcut Menu Activation? {
              n93 = event-data() -> ("CtlRef"=w286:refnum<vi>)  [unwired: 1 in]
              n94 = property class="Path"(reference=w286) -> ("Value"=w285:path)  [unwired: 1 in, 2 out]
              n95 = Empty String/Path?(string/path=w285) -> (empty?=w284:bool)
              n96 = event-data("Discard?"=w284) -> ()  [unwired: 1 in, 1 out]
            }
            event "Show ref plots window": Value Change {
              n97 = event-data() -> ("NewVal"=w287:bool)  [unwired: 1 in]
              n98 = call "Event handler-Ref plots.vi"("Show ref plots window.NewVal"=w287) -> ()  [unwired: 11 in]
            }
            event "Live stim.trig.enable", "Live stim.trig.period": Value Change {
              n99 = event-data() -> ()  [unwired: 1 in, 1 out]
              n100 = call "Stimulus trigger period event handler.vi"() -> ()  [unwired: 12 in]
            }
            event "Enable f.acq post-processing": Value Change {
              n101 = event-data() -> ("NewVal"=w288:bool)  [unwired: 1 in]
              n102 = global write "General Globals.vi" "Funct.acq post-proc enabled"(w288) -> ()
            }
            event "Live Imaging": Value Change {
              # "Sends the \" <Next state>:User Event \" case of this event structure to its specified sub-case."
              n103 = event-data() -> ("NewVal"=w293:bool)  [unwired: 1 in]
              n104 = Select(t=Top_level_VI_states."Live Imaging-START" ("event data / imaging mode"), s=w293, f=Top_level_VI_states."Live Imaging-STOP" ("event data / imaging mode")) -> (s? t:f=w291:T23)
              n105 = call "Fire User Event - Next State.vi"("\"UI Handler loop\" case to execute"=w291) -> ("Error Out"=w289:errorcluster)  [unwired: 10 in]
            }
            event "AOL Z Stack": Value Change {
              n106 = event-data() -> ("NewVal"=w295:bool)  [unwired: 1 in]
              n107 = call "Event handler-AOL Z button.vi"("AOL Z button's value"=w295) -> ("error out"=w294:errorcluster)  [unwired: 10 in]
            }
            event "Motor Z Stack": Value Change {
              n108 = event-data() -> ("NewVal"=w297:bool)  [unwired: 1 in]
              n109 = call "Event handler-Motor Z button.vi"("Motor Z button's value"=w297) -> ("error out"=w296:errorcluster)  [unwired: 10 in]
            }
            event "Funct Acq button": Value Change {
              n110 = event-data() -> ("NewVal"=w299:bool)  [unwired: 1 in]
              n111 = call "Event handler-Funct Acq button.vi"("Funct.Acq button's value"=w299) -> ("error out"=w298:errorcluster)  [unwired: 10 in]
            }
            event "Paths & Names.Base Directory": Value Change {
              n112 = event-data() -> ("OldVal"=w300:path)  [unwired: 1 in]
              n113 = call "Event handler-Dir change.vi"("Old Base Path"=w300) -> ()  [unwired: 11 in]
            }
            event "Paths & Names.User folder?": Value Change {
              n114 = event-data() -> ("NewVal"=w301:bool)  [unwired: 1 in]
              n115 = global write "General Globals.vi" "Generate user folder?"(w301) -> ()
            }
            event "Time Lapse": Value Change {
              n116 = event-data() -> ()  [unwired: 1 in, 1 out]
              n117 = call "Event handler-Time series.vi"() -> ("error out"=w302:errorcluster)  [unwired: 11 in]
            }
            event "Enable Video Recording": Value Change {
              n118 = event-data() -> ("NewVal"=w303:bool)  [unwired: 1 in]
              n119 = call "Event handler-VidRec enable.vi"("Enable Video Recording.NewVal"=w303) -> ()  [unwired: 11 in]
            }
            event "Video Record-Live Imaging": Value Change {
              n120 = event-data() -> ("NewVal"=w304:bool)  [unwired: 1 in]
              n121 = call "Event handler-VidRec enable in time series.vi"("Video Record-Live Imaging.NewVal"=w304) -> ()  [unwired: 11 in]
            }
            event "Video Record-Funct acq": Value Change {
              n122 = event-data() -> ("NewVal"=w305:bool)  [unwired: 1 in]
              n123 = call "Event handler-VidRec enable in funct.vi"("Video Record-Funct acq.NewVal"=w305) -> ()  [unwired: 11 in]
            }
            event Value Change {
              n124 = event-data() -> ("NewVal"=w306:T17)  [unwired: 1 in]
              n125 = call "fgv_AVI_Globals.vi"("AVI mode"=w306, "Function"=enum16{"Intialize", "Write", "Read", "Clear"}."Write", "\"Write\" sub function"=T25."Write AVI mode" ("\"Write\" sub function")) -> ()  [unwired: 9 in, 4 out]
            }
            event "Snapshot": Value Change {
              # "Warning! Redundant case. Eliminate if no longer needed."
              n126 = event-data() -> ()  [unwired: 1 in, 1 out]
              n127 = disable-structure shown="Disabled" {
                frame Disabled {
                  # "Right graph data"
                  # "Left graph data"
                  # "As soon as this button is pressed this code grabs both the left and right graph data (each being a 2D array of points) and saves it to the file specified by the user in a pop up file-dialogue window."
                  n128 = call "Intensity Graphs to Excel.vi"() -> ()  [unwired: 12 in]
                }
                frame Enabled {
                }
              }
            }
            event "Obtain Z Start", "Obtain Z Stop", "Z Step", "Z Start", "Z Stop": Value Change {
              n129 = event-data() -> ()  [unwired: 1 in, 1 out]
              n130 = call "Event handler-Z Setup.vi"("Obtain Z Stop"="Obtain Z Stop", "Obtain Z Start"="Obtain Z Start") -> ()  [unwired: 9 in, 1 out]
            }
            event "Pockels@Z Start", "Pockels@Z Stop": Value Change {
              n131 = event-data() -> ()  [unwired: 1 in, 1 out]
              n132 = call "Event handler-Z Setup pockels entry.vi"() -> ()  [unwired: 11 in, 1 out]
            }
            event "# Planes": Value Change {
              n133 = event-data() -> ()  [unwired: 1 in, 1 out]
              n134 = call "Event handler-Number of planes change.vi"() -> ()  [unwired: 11 in, 1 out]
            }
            event "Averages": Value Change {
              n135 = event-data() -> ("NewVal"=w311:u16)  [unwired: 1 in]
              n136 = call "Event handler-Averages ValChange.vi"("Averages.NewVal"=w311) -> ()  [unwired: 11 in]
            }
            event "AOL Z", "Zoom", "X centre", "Y centre", "Angle (degrees)", "Field of View": Value Change {
              n137 = event-data() -> ("CtlRef"=w312:refnum<vi>)  [unwired: 1 in, 2 out]
              n138 = call "Event handler-Ctrl value change.vi"("Control in"=w312) -> ()  [unwired: 11 in]
            }
            event "Dwell Time": Value Change {
              n139 = event-data() -> ()  [unwired: 1 in, 1 out]
              n140 = call "AOL Globals Dwell Time updater.vi"() -> ()  [unwired: 11 in, 1 out]
            }
            event Value Change {
              n141 = event-data() -> ()  [unwired: 1 in, 1 out]
              n142 = call "AOL Globals mode updater.vi"() -> ("error out"=w313:errorcluster)  [unwired: 11 in]
              n143 = call "AOL Globals Dwell Time updater.vi"("error in"=w313) -> ()  [unwired: 10 in, 1 out]
            }
            event "Set as Origin": Value Change {
              n144 = event-data() -> ()  [unwired: 1 in, 1 out]
              n145 = call "Event handler-Set coordinates to zero.vi"() -> ()  [unwired: 12 in]
            }
            event "Hard Shutter": Value Change {
              n146 = event-data() -> ()  [unwired: 1 in, 1 out]
              n147 = Select(t=Shutter_Function_Enum."Open Shutter" ("Shutter Function"), s="Hard Shutter", f=Shutter_Function_Enum."Close Shutter" ("Shutter Function")) -> (s? t:f=w315:T26)
              n148 = call "Set Hard Shutter.vi"("Shutter Function"=w315) -> ("Error Out"=w314:errorcluster)  [unwired: 10 in]
              n149 = case shown="Error" w314 {
                selector: w314 -> [_ w320]
                frame No Error {
                }
                frame Error {
                  w321 = T34 0 items=["no dialog", "OK message", "continue or stop message", "OK message + warnings", "continue/stop + warnings"] ("type of dialog (OK msg:1)")
                  n150 = call <vilib>:"Simple Error Handler.vi"("type of dialog (OK msg:1)"=w321, "error in (no error)"=w320) -> ("error out"=w319:errorcluster)  [unwired: 3 in, 4 out]
                  n151 = call "Window-Error message.vi"("error in (no error)"=w319, "Message"="Hard shutter error") -> ()  [unwired: 9 in, 1 out]
                }
              }
            }
            event Value Change {
              n152 = event-data() -> ("NewVal"=w323:T8)  [unwired: 1 in]
              n153 = call "Event handler-Laser power value change.vi"("Laser Power knob.NewVal"=w323) -> ()  [unwired: 11 in]
            }
            event Mouse Up; Mouse Leave {
              n154 = event-data() -> ()  [unwired: 1 in, 1 out]
              n155 = local read "Laser Power"() -> (w325:T8)
              n156 = To Unsigned Byte Integer(number=w325) -> (unsigned 8bit integer=w324:u8)
              n157 = call "Set laser power.vi"("Laser power %"=w324) -> ()  [unwired: 10 in, 1 out]
            }
            event "Ref Laser Power": Value Change {
              # "This case forces the reference frame laser power to be picked up from the \"Ref Laser Power\" control (during functional acquisition)."
              n158 = event-data() -> ()  [unwired: 1 in, 1 out]
              n159 = call "Event handler-Ref laser power change.vi"("Ref Laser Power"="Ref Laser Power") -> ()  [unwired: 11 in]
            }
            event "Funct. Acq. Pockels Modulation": Value Change {
              n160 = event-data() -> ()  [unwired: 1 in, 1 out]
              n161 = global write "gl_Pockels control globals.vi" "Funct. acq. pockels modulation?"("Funct. Acq. Pockels Modulation") -> ()
            }
            event "Virtual Shutter": Value Change {
              n162 = event-data() -> ("NewVal"=w328:bool)  [unwired: 1 in]
              n163 = call "Event handler-Virtual shutter change.vi"("Virtual shutter button value"=w328) -> ()  [unwired: 11 in]
            }
            event Value Change {
              n164 = event-data() -> ()  [unwired: 1 in, 1 out]
              n165 = call "Event handler-PMT value change.vi"() -> ()  [unwired: 12 in]
            }
            event Value Change {
              # "VI ref coming from HW config\n[SP:22-03-2018]"
              n166 = event-data() -> ()  [unwired: 1 in, 1 out]
              n167 = call "fgv_MovCor setup.vi"("Status"=enum16{"Initialize", "Write", "Read"}."Write", "MovCor Cluster"="MovCor Cluster") -> ("error out"=w330:errorcluster)  [unwired: 8 in, 1 out]
              n168 = call "Set_Ref_Parameters.vi"("error in"=w330, "use_increment_halfrate"=FALSE) -> ()  [unwired: 7 in, 3 out]
            }
            event Value Change {
              n169 = event-data() -> ()  [unwired: 1 in, 1 out]
              n170 = disable-structure shown="Enabled" {
                disable-tunnel: "RefDAQParam" -> [w338 w339]
                frame Disabled {
                  n171 = call "fgv_RefDAQParam.vi"("Function"=enum16{"Initialize", "Write", "Read"}."Write" ("Status"), "RefDAQParam in"=w338) -> ("error out"=w334:errorcluster, "RefDAQParam"=w336:T13)  [unwired: 8 in]
                  n172 = Unbundle By Name(w336) -> ("Ref_dwellTime"=w335:sgl)
                  n173 = call "Update ref dwell.vi"("error in (no error)"=w334, "Ref_dwellTime"=w335) -> ()  [unwired: 9 in, 1 out]
                }
                frame Enabled {
                  n174 = call "Update RefDAQ Parameters.vi"("RefDAQParam"=w339) -> ()  [unwired: 13 in, 2 out]
                }
              }
            }
            event "Target time between mov.cor. ref triggers (ms)": Value Change {
              n175 = event-data() -> ()  [unwired: 1 in, 1 out]
              n176 = global write "gl_Pockels control globals.vi" "Target time between mov.cor. ref triggers (ms)"("Target time between mov.cor. ref triggers (ms)") -> ()
            }
            event Value Change {
              n177 = event-data() -> ()  [unwired: 1 in, 1 out]
              n178 = call "fgv_XYStage_Move.vi"("Status"=enum16{"Initialize", "Write", "Read"}."Write", "XY Stage Move"="XY Stage Move") -> ()  [unwired: 9 in, 1 out]
            }
            event "Load Reference Image": Value Change {
              n179 = event-data() -> ()  [unwired: 1 in, 1 out]
              n180 = call "Event handler-Load ref image.vi"() -> ("error out"=w343:errorcluster)  [unwired: 10 in, 1 out]
            }
            event "Movement Correction": Value Change {
              n181 = event-data() -> ("NewVal"=w345:bool)  [unwired: 1 in]
              n182 = call "Event handler-MovCor.vi"("Movement Correction ON?"=w345, "UI queue in"=w346) -> ("error out"=w344:errorcluster)  [unwired: 9 in]
            }
            event "Axial MC": Value Change {
              n183 = event-data() -> ()  [unwired: 1 in, 3 out]
              n184 = global write "General Globals.vi" "Axial Scanning"("Axial MC") -> ()
            }
            event "Speed Logging": Value Change {
              n185 = event-data() -> ("NewVal"=w348:bool)  [unwired: 1 in]
              n186 = global write "General Globals.vi" "Speed logging enabled"(w348) -> ()
            }
            event "Motor E-Stop": Value Change {
              n187 = event-data() -> ()  [unwired: 1 in, 1 out]
              n188 = disable-structure shown="Disabled" {
                frame Disabled {
                  n189 = Bundle By Name(cluster=T27 {"Command"=enum."Initialize", "Channel"="Z", "X"=0.0, "Y"=0.0, "Z"=0.0, "Speed"=0, "Zero"=FALSE, "Use acknowledgement?"=FALSE} ("XYZ Stage data to queue"), "Use acknowledgement?"=FALSE) -> (w349:T27)
                  n190 = call "XYZ Stage-Command request module.vi"("Command"=XYZ_stage_states."Stop all movement", "XYZ Stage data to queue"=w349) -> ()  [unwired: 5 in, 5 out]
                }
                frame Enabled {
                  n191 = global write "gl_XYZStage globals.vi" "Motor E-stop"(TRUE ("Motor E-stop")) -> ()
                }
              }
            }
            event "Ls1 Confirm Wav": Value Change {
              n192 = event-data() -> ()  [unwired: 1 in, 6 out]
              n193 = call "monitor wavelength change.vi"("Actions"=T24."Stop") -> ("error out"=w355:errorcluster)  [unwired: 8 in, 2 out]
              n194 = call "FGV_Ls1 Available.vi"("FGV Actions"=enum16{"Get", "Set"}."Get", "error in (no error)"=w355) -> ("error out"=w356:errorcluster, "Laser Available ? OUT"=w357:bool)  [unwired: 8 in]
              n195 = case shown="False" w357 {
                tunnel: "Ls1 Wavelength" -> [w360 w381]
                tunnel: w356 -> [w363 w377]
                frame False {
                  n196 = call "Find Pockels calibration for wavelength.vi"("error in (no error)"=w363, "Wav"=w360) -> ("error out"=w361:errorcluster, "Ok ?"=w362:bool)  [unwired: 8 in]
                  n197 = case shown="False" w362 {
                    tunnel: w360 -> [_ w372]
                    tunnel: w361 -> [w368 w373]
                    frame False {
                      n198 = call "fgv_AOL_Globals Read.vi"("error in (no error)"=w368) -> ("error out"=w366:errorcluster, "AOL_Globals"=w367:T35)  [unwired: 8 in, 1 out]
                      n199 = Unbundle By Name(w367) -> ("Wavelength (nm)"=w365:dbl)
                      n200 = Build Array(w365) -> (w369:dbl[])
                      n201 = call "FGV user laser 1 wavelength.vi"("FGV Actions"=enum16{"Get", "Set user wavelength"}."Set user wavelength", "error in (no error)"=w366, "Laser wavelength IN"=w365) -> ()  [unwired: 7 in, 2 out]
                      n202 = call "Laser 1 FP handler L3.vi"("Numeric"=w369, "FP Ops"=Ls1_User_Ops."Update Laser Wav.", "Error in"=w366) -> ()  [unwired: 6 in, 3 out]
                    }
                    frame True {
                      n203 = call "AOL Globals wavelength updater.vi"("error in (no error)"=w373, "Laser wavelength (nm)"=w372) -> ("error out"=w371:errorcluster)  [unwired: 9 in]
                      n204 = Build Array(w372) -> (w374:dbl[])
                      n205 = call "FGV user laser 1 wavelength.vi"("FGV Actions"=enum16{"Get", "Set user wavelength"}."Set user wavelength", "Laser wavelength IN"=w372) -> ()  [unwired: 8 in, 2 out]
                      n206 = call "Laser 1 FP handler L3.vi"("Numeric"=w374, "FP Ops"=Ls1_User_Ops."Update Laser Wav.", "Error in"=w371) -> ()  [unwired: 6 in, 3 out]
                    }
                  }
                }
                frame True {
                  n207 = call "Laser wavelength change check.vi"("error in (no error)"=w377, "Laser 1 wavelength"=w381) -> ("error out"=w378:errorcluster, "Wavelength Out"=w379:u16, "Proceed ?"=w380:bool)  [unwired: 7 in]
                  n208 = case shown="True" w380 {
                    tunnel: w379 -> [_ w382]
                    tunnel: w378 -> [_ w383]
                    frame False {
                    }
                    frame True {
                      n209 = call "FGV Change laser wavelength.vi"("FGV Actions"=enum16{"Get", "Set"}."Set", "error in (no error)"=w383, "Wavelength IN"=w382, "Change Wavelength ? IN"=TRUE) -> ()  [unwired: 5 in, 3 out]
                    }
                  }
                }
              }
            }
            event "Ls1 Wavelength": Value Change {
              n210 = event-data() -> ("CtlRef"=w390:refnum<vi>, "OldVal"=w389:dbl, "NewVal"=w388:dbl)  [unwired: 1 in, 3 out]
              n211 = control-ref of="Ls1 wav cancel"() -> (w387:refnum<vi>)
              n212 = call "monitor wavelength change.vi"("Ls1 wav cancel"=w387, "Actions"=T24."Start", "new val"=w388, "Old val"=w389, "CtlRef"=w390) -> ()  [unwired: 4 in, 3 out]
            }
            event Value Change {
              n213 = event-data() -> ()  [unwired: 1 in, 6 out]
              n214 = call "monitor wavelength change.vi"("Actions"=T24."Cancel") -> ()  [unwired: 8 in, 3 out]
            }
            event "Ls1Shutter": Value Change {
              n215 = event-data() -> ()  [unwired: 1 in, 6 out]
              n216 = call "fgv_laser shutter ops.vi"("FGV Actions"=fgv_actions."Set", "Shutter state"="Ls1Shutter", "Operate Shutter"=TRUE) -> ("error out"=w392:errorcluster)  [unwired: 6 in, 2 out]
            }
            event "Generate 3D vol. images": Value Change {
              n217 = event-data() -> ()  [unwired: 1 in, 1 out]
              n218 = disable-structure shown="Disabled" {
                frame Disabled {
                  # "This functionality is only needed during development and it will be eventually eliminated."
                  n219 = call "Generate Rectangle Sequence Images.vi"("Use connector pane path input"=TRUE) -> ()  [unwired: 8 in, 3 out]
                  n220 = One Button Dialog(message="No longer available. The code module handling this was modified to handle volume imaging.") -> ()  [unwired: 1 in, 1 out]
                }
                frame Enabled {
                }
              }
            }
            event "Clear AOL GL": Value Change {
              # "This functionality is only needed during development and it will be eventually eliminated."
              n221 = event-data() -> ()  [unwired: 1 in, 1 out]
              n222 = call "fgv_AOL_Globals.vi"("Function"=enum16{"Intialize", "Write", "Read", "Clear"}."Clear") -> ()  [unwired: 9 in, 2 out]
            }
            event Value Change {
              n223 = event-data() -> ()  [unwired: 1 in, 1 out]
            }
            event "Funct. Acq. Ref frame save": Value Change {
              n224 = event-data() -> ()  [unwired: 1 in, 1 out]
              n225 = call "Message Window 2.vi"("Message string"="You must restart the software for this setting to take effect.") -> ()  [unwired: 9 in, 2 out]
            }
            event "Tracking button": Value Change {
              n226 = event-data() -> ("NewVal"=w400:bool)  [unwired: 1 in]
              n227 = case shown="True" w400 {
                frame False {
                  # "Stop tracking"
                  n228 = call "Sequence-Stop tracking.vi"() -> ()  [unwired: 11 in, 1 out]
                }
                frame True {
                  # "Start tracking"
                  n229 = call "Sequence-Start tracking.vi"() -> ()  [unwired: 12 in]
                }
              }
            }
            event "Switch user": Value Change {
              n230 = event-data() -> ()  [unwired: 1 in, 2 out]
              n231 = call "UsrProfiles-User login.vi"("Access source (Soft init)"=T31."Switch User button") -> ()  [unwired: 10 in, 1 out]
            }
            event "Abort": Value Change {
              n232 = event-data() -> ()  [unwired: 1 in, 1 out]
              n233 = call "Enqueue Message.vi"("Message"="Stop", "Queue"=w403) -> ("error out"=w402:errorcluster)  [unwired: 8 in, 1 out]
            }
            event User Event {
              # "Do not add any code in this case.\nThis case is only used to cause the event loop to stop.\nuse the subVI in the disaboled case below to fire a programmatic event from anywhere, which will stop the event handling loop."
              n234 = event-data() -> ()  [unwired: 1 in, 1 out]
              n235 = disable-structure shown="Enabled" {
                frame Disabled {
                  n236 = call "Fire User Event - Stop.vi"() -> ()  [unwired: 11 in, 1 out]
                }
                frame Enabled {
                }
              }
            }
            event "Exit button": Value Change {
              # "The UI Message Loop handles sending the Exit message to other loops."
              n237 = event-data() -> ()  [unwired: 1 in, 1 out]
              n238 = call "Event handler-Exit.vi"("UI queue"=w406) -> ("error out"=w407:errorcluster)  [unwired: 9 in, 1 out]
            }
            event Panel Close? {
              n239 = event-data() -> ()  [unwired: 1 in, 1 out]
              n240 = call "Event handler-Exit.vi"("UI queue"=w409) -> ("error out"=w410:errorcluster)  [unwired: 9 in, 1 out]
              n241 = event-data("Discard?"=TRUE) -> ()  [unwired: 1 in, 1 out]
            }
          }
          n242 = call "Event loop error handler.vi"("error in (no error)"=w274, "Next State"=w266, "Stop?"=w268) -> ("error out"=w270:errorcluster, "Stop event handling loop"=w275:bool)  [unwired: 7 in]
        }
        n243 = while {
          tunnel: w23 -> [w41]
          tunnel: w11 -> [w38]
          tunnel: [w37] -> w12
          shift-right: [w35] -> _
          shift-left: w22 -> [w40]
          tunnel: [w36] -> _
          i -> [w36]
          stop <- w45 stop-if-true
          # "UI Handler Loop"
          n244 = call "Dequeue Message.vi"("Error In"=w38, "Message Queue"=w41) -> ("Error Out"=w44:errorcluster, "Message Data"=w42:variant, "Message"=w43:string, "dup Message Queue"=w33:refnum<queue>)  [unwired: 5 in, 1 out]
          n245 = case "Message Cases" shown="\"Live Imaging\"" w43 {
            selector: w43 -> [w50 _ _ _ _ _ _ w97 w118 w139 w165 w186 w206 w226 w245]
            tunnel: w33 -> [_ w56 _ w78 _ w87 _ w106 w127 w148 w161 w194 w211 w234 w250]
            tunnel: w44 -> [_ w59 w67 w73 w80 w93 w95 w105 w126 w147 w168 w193 w213 w233 w252]
            tunnel: [w48 w52 w68 w72 w83 w91 w95 w101 w122 w143 w162 w190 w209 w231 w254] -> w39
            tunnel: [_ _ _ _ _ w92 _ _ _ _ _ _ _ _ _] -> w45
            tunnel: w42 -> [_ _ w66 _ _ _ _ w103 w124 w145 w167 w192 w214 w229 w248]
            tunnel: w40 -> [w46 w57 w62 w74 w82 w89 w94 w99 w120 w141 w164 w188 w215 w228 w247]
            tunnel: [w46 w57 w62 w71 w82 w90 w94 w98 w119 w140 w163 w187 w207 w227 w246] -> w35
            tunnel: [_ _ _ _ _ _ _ w96 w117 w138 w158 w185 w205 w224 w244] -> w34
            frame Default {
              # "'Default' case only runs if there is a message that isn't defined in any of the other cases.  Output a programming error."
              n246 = Format Into String(format string="The invalid message string \"%s\" was received in the Message Handling Loop." ("Invalid Message Loop Message"), w50) -> (resulting string=w47:string)  [unwired: 2 in, 1 out]
              n247 = call <vilib>:"Error Cluster From Error Code.vi"("error message (\"\")"=w47, "error code (0)"=1) -> ("error out"=w48:errorcluster)  [unwired: 7 in]
            }
            frame "Initialize" {
              n248 = call "Update Last State indicator value.vi"("error in (no error)"=w59, "Value"="Software Initialised") -> ("error out"=w55:errorcluster)  [unwired: 9 in]
              n249 = call "Enqueue Message.vi"("error in (no error)"=w55, "Message Data"="Ready" ("Ready..."), "Message"="Update Status", "Queue"=w56) -> ("error out"=w53:errorcluster)  [unwired: 6 in, 1 out]
              n250 = call "Ctrls state & value on Start-Stop.vi"("error in (no error)"=w53, "Queue data"=T21 {"Start/Stop"=enum."STOP", "State"=enum."Live Imaging-STOP"}) -> ("error out"=w52:errorcluster)  [unwired: 9 in]
            }
            frame "Update Status" {
              # "Update Display - Convert the message data to a string to display in the Status indicator."
              n251 = Variant To Data(error in=w67, type="", Variant=w66) -> (data=→"Status ind":string, error out=w63:errorcluster)
              n252 = Merge Errors(w63) -> (w68:errorcluster)
            }
            frame "Stop" {
              # "Stops the acquisition"
              # "Stop - Enable/Disable buttons appropriately for an acquisition that has stopped, and update status display."
              n253 = call "Enqueue Message.vi"("error in (no error)"=w73, "Message"="Stop", "Queue"=w74) -> ("error out"=w72:errorcluster, "Queue out"=w71:refnum<queue>)  [unwired: 7 in]
              n254 = call "Enqueue Message.vi"("error in (no error)"=w73, "Message Data"="Stopped" ("Ready..."), "Message"="Update Status", "Queue"=w78) -> ("error out"=w70:errorcluster)  [unwired: 6 in, 1 out]
              n255 = call <vilib>:"Clear Errors.vi"("error in (no error)"=w70) -> ("error out"=w69:errorcluster)  [unwired: 5 in, 1 out]
              n256 = call "UI Cleanup.vi"("error in (no error)"=w69) -> ()  [unwired: 10 in, 1 out]
            }
            frame "Unload subpanel" {
              # "Update Display - Convert the message data to a string to display in the Status indicator."
              n257 = global read "General Globals.vi" "Subpanel is open"() -> (w81:bool)
              n258 = invoke on="Sub Panel" class="SubPnl" method="Remove VI"(error in=w80) -> (error out=w79:errorcluster)  [unwired: 2 in, 2 out]
              n259 = case shown="True" w81 {
                tunnel: w79 -> [w84 w86]
                tunnel: [w84 w86] -> w83
                frame False {
                }
                frame True {
                  # "A subpanel is open"
                  n260 = global write "General Globals.vi" "Stop subpanel"(TRUE ("Stop subpanel")) -> ()
                }
              }
            }
            frame "Exit" {
              w92 = TRUE
              # "Exit - Fire the User Event to stop the Event Handling Loop.  Also send Exit messages to the Acqusition and Logging loops."
              n261 = call "Exit case.vi"("error in"=w93, "UI queue"=w87, "Acq. queue"=w89) -> ("error out"=w91:errorcluster, "Exit String"=w88:string, "Acq. queue (out)"=w90:refnum<queue>)  [unwired: 6 in]
              n262 = local write "Status ind"(w88) -> ()
              "Stop" <- w92
            }
            frame "<IMAGING CASES BELOW>" {
            }
            frame "AOL Z Stack" {
              n263 = call "Variant to Data-Imaging protocol queue.vi"("error in (no error)"=w105, "Message Data"=w103) -> ("error out"=w104:errorcluster, "Next state queue data"=w96:T21)  [unwired: 8 in]
              n264 = Unbundle By Name(w96) -> ("Start/Stop"=w102:T22)
              n265 = case shown="\"START\"" w102 {
                tunnel: w106 -> [w107 _]
                tunnel: w104 -> [w108 w116]
                tunnel: w99 -> [w112 w115]
                tunnel: [w110 w116] -> w100
                tunnel: [w111 w115] -> w98
                tunnel: w97 -> [w109 _]
                frame "START" {
                  n266 = call "Start Logic.vi"("error in (no error)"=w108, "Case name string"=w109, "UI queue"=w107, "Acq. queue in"=w112) -> ("error out"=w110:errorcluster, "Acq. queue"=w111:refnum<queue>)  [unwired: 6 in]
                }
                frame "STOP", Default {
                  # "Place here (as a sub-VI) any code that you need to execute when the \"AOL Z Stack\" completes.\nUse the \"Fire User Event - Next State.vi\" to fire a programatic event and cause this case to execute."
                  n267 = call "Pockels-manage mod setting.vi"("Function"=enum16{"Capture setting", "Re-apply setting"}."Re-apply setting") -> ()  [unwired: 10 in, 1 out]
                  n268 = call "Set MC Test Data Global.vi"("Save MC TestData"=FALSE) -> ()  [unwired: 9 in, 2 out]
                }
              }
              n269 = call "Ctrls state & value on Start-Stop.vi"("error in (no error)"=w100, "Queue data"=w96) -> ("error out"=w101:errorcluster)  [unwired: 9 in]
            }
            frame "Parameter Sweep" {
              n270 = call "Variant to Data-Imaging protocol queue.vi"("error in (no error)"=w126, "Message Data"=w124) -> ("error out"=w125:errorcluster, "Next state queue data"=w117:T21)  [unwired: 8 in]
              n271 = Unbundle By Name(w117) -> ("Start/Stop"=w123:T22)
              n272 = case shown="\"START\"" w123 {
                tunnel: w127 -> [w128 _]
                tunnel: w125 -> [w129 w137]
                tunnel: w120 -> [w133 w136]
                tunnel: [w131 w137] -> w121
                tunnel: [w132 w136] -> w119
                tunnel: w118 -> [w130 _]
                frame "START" {
                  n273 = call "Start Logic.vi"("error in (no error)"=w129, "Case name string"=w130, "UI queue"=w128, "Acq. queue in"=w133) -> ("error out"=w131:errorcluster, "Acq. queue"=w132:refnum<queue>)  [unwired: 6 in]
                }
                frame "STOP", Default {
                  # "Place here (as a sub-VI) any code that you need to execute when the \"AOL Z Stack\" completes.\nUse the \"Fire User Event - Next State.vi\" to fire a programatic event and cause this case to execute."
                  n274 = call "Pockels-manage mod setting.vi"("Function"=enum16{"Capture setting", "Re-apply setting"}."Re-apply setting") -> ()  [unwired: 10 in, 1 out]
                  n275 = call "Set MC Test Data Global.vi"("Save MC TestData"=FALSE) -> ()  [unwired: 9 in, 2 out]
                }
              }
              n276 = call "Ctrls state & value on Start-Stop.vi"("error in (no error)"=w121, "Queue data"=w117) -> ("error out"=w122:errorcluster)  [unwired: 9 in]
            }
            frame "Motor Z Stack" {
              n277 = call "Variant to Data-Imaging protocol queue.vi"("error in (no error)"=w147, "Message Data"=w145) -> ("error out"=w146:errorcluster, "Next state queue data"=w138:T21)  [unwired: 8 in]
              n278 = Unbundle By Name(w138) -> ("Start/Stop"=w144:T22)
              n279 = case shown="\"STOP\", Default" w144 {
                tunnel: [w151 w153] -> w142
                tunnel: w141 -> [w150 w157]
                tunnel: w148 -> [_ w155]
                tunnel: w146 -> [w151 w152]
                tunnel: [w150 w156] -> w140
                tunnel: w139 -> [_ w154]
                frame "STOP", Default {
                  # "Place here (as a sub-VI) any code that you need to execute when the \"Motor Z Stack\" completes.\nUse the \"Fire User Event - Next State.vi\" to fire a programatic event and cause this case to execute."
                  n280 = call "Pockels-manage mod setting.vi"("Function"=enum16{"Capture setting", "Re-apply setting"}."Re-apply setting") -> ()  [unwired: 10 in, 1 out]
                }
                frame "START" {
                  n281 = call "Start Logic.vi"("error in (no error)"=w152, "Case name string"=w154, "UI queue"=w155, "Acq. queue in"=w157) -> ("error out"=w153:errorcluster, "Acq. queue"=w156:refnum<queue>)  [unwired: 6 in]
                }
              }
              n282 = call "Ctrls state & value on Start-Stop.vi"("error in (no error)"=w142, "Queue data"=w138) -> ("error out"=w143:errorcluster)  [unwired: 9 in]
            }
            frame "Live Imaging" {
              n283 = call "Variant to Data-Imaging protocol queue.vi"("error in (no error)"=w168, "Message Data"=w167) -> ("error out"=w160:errorcluster, "Next state queue data"=w158:T21)  [unwired: 8 in]
              n284 = call "Ctrls state & value on Start-Stop.vi"("error in (no error)"=w160, "Queue data"=w158) -> ("error out"=w159:errorcluster)  [unwired: 9 in]
              n285 = Unbundle By Name(w158) -> ("Start/Stop"=w166:T22)
              n286 = case shown="\"START\"" w166 {
                tunnel: w164 -> [w173 w180]
                tunnel: [w170 w183] -> w162
                tunnel: w161 -> [w172 w179]
                tunnel: w159 -> [w171 w182]
                tunnel: w165 -> [_ w178]
                tunnel: [w173 w181] -> w163
                frame "STOP", Default {
                  n287 = call "Stop Logic-Imaging.vi"("error in (no error)"=w171, "UI queue"=w172) -> ("error out"=w169:errorcluster)  [unwired: 9 in]
                  n288 = disable-structure shown="Enabled" {
                    disable-tunnel: [w176 w177] -> w170
                    disable-tunnel: w169 -> [w175 w177]
                    frame Disabled {
                      n289 = call "Set MC Test Data Global.vi"("error in (no error)"=w175, "Save MC TestData"=FALSE) -> ("error out"=w176:errorcluster)  [unwired: 8 in, 1 out]
                    }
                    frame Enabled {
                    }
                  }
                }
                frame "START" {
                  n290 = call "Start Logic.vi"("error in (no error)"=w182, "Case name string"=w178, "UI queue"=w179, "Acq. queue in"=w180) -> ("error out"=w183:errorcluster, "Acq. queue"=w181:refnum<queue>)  [unwired: 6 in]
                }
              }
            }
            frame "Live volume imaging" {
              n291 = call "Variant to Data-Imaging protocol queue.vi"("error in (no error)"=w193, "Message Data"=w192) -> ("error out"=w184:errorcluster, "Next state queue data"=w185:T21)  [unwired: 8 in]
              n292 = Unbundle By Name(w185) -> ("Start/Stop"=w191:T22)
              n293 = case shown="\"START\"" w191 {
                tunnel: w194 -> [w195 w202]
                tunnel: w188 -> [w198 w204]
                tunnel: [w196 w199] -> w189
                tunnel: w184 -> [w197 w201]
                tunnel: [w198 w203] -> w187
                tunnel: w186 -> [_ w200]
                frame "STOP", Default {
                  n294 = call "Stop Logic-Imaging.vi"("error in (no error)"=w197, "UI queue"=w195) -> ("error out"=w196:errorcluster)  [unwired: 9 in]
                }
                frame "START" {
                  n295 = call "Start Logic.vi"("error in (no error)"=w201, "Case name string"=w200, "UI queue"=w202, "Acq. queue in"=w204) -> ("error out"=w199:errorcluster, "Acq. queue"=w203:refnum<queue>)  [unwired: 6 in]
                }
              }
              n296 = call "Ctrls state & value on Start-Stop.vi"("error in (no error)"=w189, "Queue data"=w185) -> ("error out"=w190:errorcluster)  [unwired: 9 in]
            }
            frame "Functional Acquisition" {
              n297 = call "Variant to Data-Imaging protocol queue.vi"("error in (no error)"=w213, "Message Data"=w214) -> ("error out"=w212:errorcluster, "Next state queue data"=w205:T21)  [unwired: 8 in]
              n298 = Unbundle By Name(w205) -> ("Start/Stop"=w210:T22)
              n299 = case shown="\"START\"" w210 {
                tunnel: w215 -> [w221 w222]
                tunnel: [w217 w223] -> w208
                tunnel: w212 -> [w216 w223]
                tunnel: w211 -> [w219 _]
                tunnel: [w220 w222] -> w207
                tunnel: w206 -> [w218 _]
                frame "START" {
                  n300 = call "Start Logic.vi"("error in (no error)"=w216, "Case name string"=w218, "UI queue"=w219, "Acq. queue in"=w221) -> ("error out"=w217:errorcluster, "Acq. queue"=w220:refnum<queue>)  [unwired: 6 in]
                }
                frame "STOP", Default {
                  n301 = call "Funct Acq Stop Actions.vi"() -> ()  [unwired: 12 in]
                }
              }
              n302 = call "Ctrls state & value on Start-Stop.vi"("error in (no error)"=w208, "Queue data"=w205) -> ("error out"=w209:errorcluster)  [unwired: 9 in]
            }
            frame "Single Plane Acquisition" {
              n303 = call "Variant to Data-Imaging protocol queue.vi"("error in (no error)"=w233, "Message Data"=w229) -> ("error out"=w232:errorcluster, "Next state queue data"=w224:T21)  [unwired: 8 in]
              n304 = Unbundle By Name(w224) -> ("Start/Stop"=w230:T22)
              n305 = case shown="\"START\"" w230 {
                tunnel: w234 -> [w238 _]
                tunnel: w228 -> [w240 w242]
                tunnel: w232 -> [w236 w243]
                tunnel: [w239 w242] -> w227
                tunnel: w226 -> [w237 _]
                tunnel: [w235 w243] -> w225
                frame "START" {
                  n306 = call "Start Logic.vi"("error in (no error)"=w236, "Case name string"=w237, "UI queue"=w238, "Acq. queue in"=w240) -> ("error out"=w235:errorcluster, "Acq. queue"=w239:refnum<queue>)  [unwired: 6 in]
                }
                frame "STOP", Default {
                  # "Place here (as a sub-VI) any code that you need to execute when the \"Single Plane Acquitition\" completes.\nUse the \"Fire User Event - Next State.vi\" to fire a programatic event and cause this case to execute."
                  n307 = call "Pockels-manage mod setting.vi"("Function"=enum16{"Capture setting", "Re-apply setting"}."Re-apply setting") -> ()  [unwired: 10 in, 1 out]
                }
              }
              n308 = call "Ctrls state & value on Start-Stop.vi"("error in (no error)"=w225, "Queue data"=w224) -> ("error out"=w231:errorcluster)  [unwired: 9 in]
            }
            frame "Volume acquisition" {
              n309 = call "Variant to Data-Imaging protocol queue.vi"("error in (no error)"=w252, "Message Data"=w248) -> ("error out"=w251:errorcluster, "Next state queue data"=w244:T21)  [unwired: 8 in]
              n310 = Unbundle By Name(w244) -> ("Start/Stop"=w249:T22)
              n311 = case shown="\"STOP\", Default" w249 {
                tunnel: w247 -> [w259 w263]
                tunnel: [w257 w264] -> w253
                tunnel: w251 -> [w260 w264]
                tunnel: w250 -> [w256 _]
                tunnel: [w258 w263] -> w246
                tunnel: w245 -> [w255 _]
                frame "START" {
                  n312 = call "Start Logic.vi"("error in (no error)"=w260, "Case name string"=w255, "UI queue"=w256, "Acq. queue in"=w259) -> ("error out"=w257:errorcluster, "Acq. queue"=w258:refnum<queue>)  [unwired: 6 in]
                }
                frame "STOP", Default {
                  # "Place here (as a sub-VI) any code that you need to execute when the \"Volume acquisition\" completes.\nUse the \"Fire User Event - Next State.vi\" to fire a programatic event and cause this case to execute."
                  n313 = call "Set MC Test Data Global.vi"("Save MC TestData"=FALSE) -> ()  [unwired: 9 in, 2 out]
                  n314 = call "Pockels-manage mod setting.vi"("Function"=enum16{"Capture setting", "Re-apply setting"}."Re-apply setting") -> ()  [unwired: 10 in, 1 out]
                }
              }
              n315 = call "Ctrls state & value on Start-Stop.vi"("error in (no error)"=w253, "Queue data"=w244) -> ("error out"=w254:errorcluster)  [unwired: 9 in]
            }
          }
          n316 = call "Error handler-UI handling loop.vi"("error in (no error)"=w39) -> ("No error"=w37:errorcluster)  [unwired: 10 in]
          n317 = call "Set status to Idle.vi"("Next state queue data"=w34, "UI queue"=w33) -> ()  [unwired: 10 in]
        }
        n318 = Unregister For Events(event registration refnum=w25) -> (error out=w14:errorcluster)  [unwired: 1 in]
        n319 = call "Compute Chirp Parameters.vi"("Error in"=w10) -> ("error out"=w18:errorcluster)  [unwired: 9 in, 1 out]
        n320 = call "Utility processes.vi"("error in (no error)"=w10) -> ("error out"=w9:errorcluster)  [unwired: 10 in]
        n321 = call "Acquisition Module.vi"("Error In"=w10, "Queues Cluster"=w7) -> ("Error Out"=w17:errorcluster)  [unwired: 9 in]
        n322 = call "Logging Module.vi"("Logging process enabled"=TRUE, "Data Queue error in"=w10, "Queues Cluster"=w7) -> ("error out"=w21:errorcluster)  [unwired: 8 in]
        n323 = call "Encoder Driver.vi"("UI elements cluster"=w5) -> ("Error out (no error)"=w20:errorcluster)  [unwired: 10 in]
        n324 = call "XYZ Stage Driver (ver 2).vi"("UI elements cluster"=w5) -> ("error out (no error)"=w6:errorcluster)  [unwired: 10 in]
        n325 = call "Laser 1 Operations L3.vi"("UI elements cluster"=w5) -> ("Error out"=w8:errorcluster)  [unwired: 10 in]
        n326 = call <vilib>:"Clear Errors.vi"("error in (no error)"=w14) -> ()  [unwired: 5 in, 2 out]
        n327 = Merge Errors(w15, w12, w18, w9, w17, w21, w20, w6, w8) -> (w19:errorcluster)
        n328 = call "Software Cleanup.vi"("error in (no error)"=w19) -> ("error out"=w16:errorcluster)  [unwired: 10 in]
        n329 = flat-sequence {
          tunnel: w16 -> [_]
          tunnel: [w29] -> w26
          frame #0 {
            n330 = global read "General Globals.vi" "Restart"() -> (w29:bool)
            n331 = Request Deallocation(TRUE ("flag")) -> ()
          }
        }
        n332 = case shown="False" w26 {
          frame False {
            n333 = call "Close panel if exe-Top level VI.vi"() -> ()  [unwired: 11 in, 1 out]
          }
          frame True {
            # "Probably not\nneeded"
            n334 = Wait (ms)(milliseconds to wait=u32 1000) -> ()  [unwired: 1 out]
          }
        }
      }
      frame True {
        # "Application shutting down due to lack of admin proviledges"
        n335 = global write "gl_UI Ctrl Refs.vi" "UI ctrl refs"(w411) -> ()
        n336 = flat-sequence {
          tunnel: w411 -> [_]
          frame #0 {
            n337 = call "Close panel if exe-Top level VI.vi"() -> ()  [unwired: 11 in, 1 out]
          }
        }
      }
    }
  }
